vi "Durability Tank Cal UI.vi"(11 "Calling VI Ref":refnum<vi>) -> ()   [LabVIEW 2013]
uses:
  <vilib>/ptbypt/NI_PtbyPt.lvlib
  <vilib>/Utility/file.llb/Read From Spreadsheet File (string).vi
  <vilib>/Utility/miscctls.llb/LVRowAndColumnTypeDef.ctl
  <vilib>/Analysis/NI_AALPro.lvlib
  <resource>/objmgr/daqmx.rc
  Type Defs/Target Cluster Type Def.ctl
  Type Defs/Setpoint Cluster Type Def.ctl
  Type Defs/Targets Type Def.ctl
  <vilib>/Utility/config.llb/NI_LVConfig.lvlib
  Type Defs/Units Type Def (DAQ Rack).ctl
  Type Defs/Rack Version Type Def.ctl
  <userlib>/_OpenG.lib/array/array.llb/Remove Duplicates from 1D Array (DBL)__ogtk.vi
  <vilib>/Utility/file.llb/Write To Spreadsheet File (string).vi
  <vilib>/DAQmx/write.llb/DAQmx Write (Digital Bool 1Line 1Point).vi
  <vilib>/DAQmx/create/channels.llb/DAQmx Create Channel (DO-Digital Output).vi
  <vilib>/DAQmx/write.llb/DAQmx Write (Digital 1D Bool NChan 1Samp 1Line).vi
  <userlib>/_OpenG.lib/array/array.llb/Search 1D Array (String)__ogtk.vi
  Type Defs/System Type.ctl
  Type Defs/Registered System.ctl
  Type Defs/TCP Data Stream Mode (PC).ctl
  Type Defs/Channel Type Def (RIO).ctl
panel:
  in  "App Dir":path
  in  "Load Indicator Tab":enum32{"Page 1"}(tab)
  in  "Header Tab":enum32{"Page 1", "Page 2"}(tab)
  in  "Header OK":bool
  in  "Header Cancel":bool
  in  "Header Comments":string[][](table)=[["PRODUCT 5V. IS REFERENCE ONLY."], ["1"], ["2"]]
  in  "Cal Standards Table":string[][](table)=[["FLUKE MULTIMETER", "3539"], ["FLUKE CALIBRATOR", "7955"], ["", ""], ["", ""], ["", ""]]
  in  "Sys Cal Table":string[][](table)=[["CIB BD.", "DSS 9372-1"], ["D/A BD.", "DSS 9372-2"], ["", ""], ["", ""], ["", ""]]
  in  "Header Table 1":string[][](table)=[["9372blah"], ["DELPHI"], ["TL1181E"], ["EU2C397"], ["CIB/ D/A BD."], ["5 VOLTS"], ["NEW"], ["9087"]]
  in  "Header Table 2":string[][](table)=[["39687"], ["12"], ["40052"], ["MDC"], ["24"], ["48"], ["JUM  /   DR"]]
  in  "debug":bool=TRUE
  in  "Verify Tab":enum32{"Page 1", "Page 2"}(tab)
  in  "Hide Devs":bool
  in  "Auto":bool
  in  "Hide Cal Values":bool
  in  "Verify Edit":bool
  in  "Verify Table":string[][](table)=[["", "0", "0"], ["", "3", "3"], ["", "6", "6"], ["", "9", "9"], ["", "12", "12"], ["", "15", "15"], ["", "", ""], ["", "", ""], ["", "", ""], ["", "", ""]]
  in  "Verify Read":bool
  in  "ms":u32=1000
  in  "avg":i32=5
  in  "Output Tab":enum32{"Page 1", "Page 2"}(tab)
  out "Row":i32
  in  "Main Tab":enum32{"Page 1", "Page 2"}(tab)
  in  "Confirm 4th Point":bool
  out "Reading Value 4":dbl=0.001 caption="reading" format="%#.4g"
  in  "Cal Value 4":dbl caption="cal pt" format="%#.4g"
  in  "Confirm 5th Point":bool
  out "Reading Value 5":dbl=0.0016 caption="reading" format="%#.4g"
  in  "Cal Value 5":dbl caption="cal pt" format="%#.4g"
  in  "Start Verification":bool
  in  "View Spreadsheet":bool
  in  "Header":bool
  out "Cal Table":string[][](table)=[["AI-00", "V", "", "", "", "", "", "", "", "", "", "", "", "", "", "", "", "", "", "", "", "", "", "", "", "", "", "", "", "", "", ""], ["AI-01", "V", "", "", "", "", "", "", "", "", "", "", "", "", "", "", "", "", "", "", "", "", "", "", "", "", "", "", "", "", "", ""], ["AI-02", "V", "", "", "", "", "", "", "", "", "", "", "", "", "", "", "", "", "", "", "", "", "", "", "", "", "", "", "", "", "", ""], ["AI-03", "V", "", "", "", "", "", "", "", "", "", "", "", "", "", "", "", "", "", "", "", "", "", "", "", "", "", "", "", "", "", ""], ["AI-04", "V", "", "", "", "", "", "", "", "", "", "", "", "", "", "", "", "", "", "", "", "", "", "", "", "", "", "", "", "", "", ""], ["AI-05", "V", "", "", "", "", "", "", "", "", "", "", "", "", "", "", "", "", "", "", "", "", "", "", "", "", "", "", "", "", "", ""], ["AI-06", "V", "", "", "", "", "", "", "", "", "", "", "", "", "", "", "", "", "", "", "", "", "", "", "", "", "", "", "", "", "", ""], ["AI-07", "V", "", "", "", "", "", "", "", "", "", "", "", "", "", "", "", "", "", "", "", "", "", "", "", "", "", "", "", "", "", ""], ["AI-08", "V", "", "", "", "", "", "", "", "", "", "", "", "", "", "", "", "", "", "", "", "", "", "", "", "", "", "", "", "", "", ""], ["AI-09", "V", "", "", "", "", "", "", "", "", "", "", "", "", "", "", "", "", "", "", "", "", "", "", "", "", "", "", "", "", "", ""], ["AI-10", "V", "", "", "", "", "", "", "", "", "", "", "", "", "", "", "", "", "", "", "", "", "", "", "", "", "", "", "", "", "", ""], ["AI-11", "V", "", "", "", "", "", "", "", "", "", "", "", "", "", "", "", "", "", "", "", "", "", "", "", "", "", "", "", "", "", ""], ["AI-12", "V", "", "", "", "", "", "", "", "", "", "", "", "", "", "", "", "", "", "", "", "", "", "", "", "", "", "", "", "", "", ""], ["AI-13", "V", "", "", "", "", "", "", "", "", "", "", "", "", "", "", "", "", "", "", "", "", "", "", "", "", "", "", "", "", "", ""], ["AI-14", "V", "", "", "", "", "", "", "", "", "", "", "", "", "", "", "", "", "", "", "", "", "", "", "", "", "", "", "", "", "", ""], ["AI-15", "V", "", "", "", "", "", "", "", "", "", "", "", "", "", "", "", "", "", "", "", "", "", "", "", "", "", "", "", "", "", ""], ["AI-16", "V", "", "", "", "", "", "", "", "", "", "", "", "", "", "", "", "", "", "", "", "", "", "", "", "", "", "", "", "", "", ""], ["AI-17", "V", "", "", "", "", "", "", "", "", "", "", "", "", "", "", "", "", "", "", "", "", "", "", "", "", "", "", "", "", "", ""], ["AI-18", "V", "", "", "", "", "", "", "", "", "", "", "", "", "", "", "", "", "", "", "", "", "", "", "", "", "", "", "", "", "", ""], ["AI-19", "V", "", "", "", "", "", "", "", "", "", "", "", "", "", "", "", "", "", "", "", "", "", "", "", "", "", "", "", "", "", ""], ["AI-20", "V", "", "", "", "", "", "", "", "", "", "", "", "", "", "", "", "", "", "", "", "", "", "", "", "", "", "", "", "", "", ""], ["AI-21", "V", "", "", "", "", "", "", "", "", "", "", "", "", "", "", "", "", "", "", "", "", "", "", "", "", "", "", "", "", "", ""], ["AI-22", "V", "", "", "", "", "", "", "", "", "", "", "", "", "", "", "", "", "", "", "", "", "", "", "", "", "", "", "", "", "", ""], ["AI-23", "V", "", "", "", "", "", "", "", "", "", "", "", "", "", "", "", "", "", "", "", "", "", "", "", "", "", "", "", "", "", ""], ["AI-24", "V", "", "", "", "", "", "", "", "", "", "", "", "", "", "", "", "", "", "", "", "", "", "", "", "", "", "", "", "", "", ""], ["AI-25", "V", "", "", "", "", "", "", "", "", "", "", "", "", "", "", "", "", "", "", "", "", "", "", "", "", "", "", "", "", "", ""], ["AI-26", "V", "", "", "", "", "", "", "", "", "", "", "", "", "", "", "", "", "", "", "", "", "", "", "", "", "", "", "", "", "", ""], ["AI-27", "V", "", "", "", "", "", "", "", "", "", "", "", "", "", "", "", "", "", "", "", "", "", "", "", "", "", "", "", "", "", ""], ["AI-28", "V", "", "", "", "", "", "", "", "", "", "", "", "", "", "", "", "", "", "", "", "", "", "", "", "", "", "", "", "", "", ""], ["AI-29", "V", "", "", "", "", "", "", "", "", "", "", "", "", "", "", "", "", "", "", "", "", "", "", "", "", "", "", "", "", "", ""], ["AI-30", "V", "", "", "", "", "", "", "", "", "", "", "", "", "", "", "", "", "", "", "", "", "", "", "", "", "", "", "", "", "", ""], ["AI-31", "V", "", "", "", "", "", "", "", "", "", "", "", "", "", "", "", "", "", "", "", "", "", "", "", "", "", "", "", "", "", ""], ["TC-00", "degF", "", "", "", "", "", "", "", "", "", "", "", "", "", "", "", "", "", "", "", "", "", "", "", "", "", "", "", "", "", ""], ["TC-01", "degF", "", "", "", "", "", "", "", "", "", "", "", "", "", "", "", "", "", "", "", "", "", "", "", "", "", "", "", "", "", ""], ["TC-02", "degF", "", "", "", "", "", "", "", "", "", "", "", "", "", "", "", "", "", "", "", "", "", "", "", "", "", "", "", "", "", ""], ["TC-03", "degF", "", "", "", "", "", "", "", "", "", "", "", "", "", "", "", "", "", "", "", "", "", "", "", "", "", "", "", "", "", ""], ["TC-04", "degF", "", "", "", "", "", "", "", "", "", "", "", "", "", "", "", "", "", "", "", "", "", "", "", "", "", "", "", "", "", ""], ["TC-05", "degF", "", "", "", "", "", "", "", "", "", "", "", "", "", "", "", "", "", "", "", "", "", "", "", "", "", "", "", "", "", ""], ["TC-06", "degF", "", "", "", "", "", "", "", "", "", "", "", "", "", "", "", "", "", "", "", "", "", "", "", "", "", "", "", "", "", ""], ["TC-07", "degF", "", "", "", "", "", "", "", "", "", "", "", "", "", "", "", "", "", "", "", "", "", "", "", "", "", "", "", "", "", ""], ["TC-08", "degF", "", "", "", "", "", "", "", "", "", "", "", "", "", "", "", "", "", "", "", "", "", "", "", "", "", "", "", "", "", ""], ["TC-09", "degF", "", "", "", "", "", "", "", "", "", "", "", "", "", "", "", "", "", "", "", "", "", "", "", "", "", "", "", "", "", ""], ["TC-10", "degF", "", "", "", "", "", "", "", "", "", "", "", "", "", "", "", "", "", "", "", "", "", "", "", "", "", "", "", "", "", ""], ["TC-11", "degF", "", "", "", "", "", "", "", "", "", "", "", "", "", "", "", "", "", "", "", "", "", "", "", "", "", "", "", "", "", ""], ["TC-12", "degF", "", "", "", "", "", "", "", "", "", "", "", "", "", "", "", "", "", "", "", "", "", "", "", "", "", "", "", "", "", ""], ["TC-13", "degF", "", "", "", "", "", "", "", "", "", "", "", "", "", "", "", "", "", "", "", "", "", "", "", "", "", "", "", "", "", ""], ["TC-14", "degF", "", "", "", "", "", "", "", "", "", "", "", "", "", "", "", "", "", "", "", "", "", "", "", "", "", "", "", "", "", ""], ["TC-15", "degF", "", "", "", "", "", "", "", "", "", "", "", "", "", "", "", "", "", "", "", "", "", "", "", "", "", "", "", "", "", ""], ["", "", "", "", "", "", "", "", "", "", "", "", "", "", "", "", "", "", "", "", "", "", "", "", "", "", "", "", "", "", "", ""]]
  out "Tank IP:":string
  in  "Start Cal":bool
  in  "Confirm 1st Point":bool
  out "Reading Value 1":dbl caption="reading" format="%#.4g"
  in  "Cal Value 1":dbl caption="cal pt" format="%#.4g"
  in  "Confirm 2nd Point":bool
  out "Reading Value 2":dbl=0.001 caption="reading" format="%#.4g"
  in  "Cal Value 2":dbl caption="cal pt" format="%#.4g"
  in  "Save Cal":bool
  out "f(x)":dbl format="%#.4g"
  out "a0":dbl format="%#.4g"
  out "x":dbl=0.0006000000000000001 format="%#.4g"
  out "a2":dbl format="%#.4g"
  in  "Cancel Cal":bool
  out "Cal Unit":T1
  in  "Confirm 3rd Point":bool
  out "Reading Value 3":dbl=0.0016 caption="reading" format="%#.4g"
  in  "Cal Value 3":dbl caption="cal pt" format="%#.4g"
  out "a1":dbl format="%#.4g"
  in  "Channel to Cal":T2
  out "a3":dbl format="%#.4g"
  out "a4":dbl format="%#.4g"
  # "System Calibration Components"
  # "Calibration Standards Used"
  # "Output Control"
  # "1) Enter Header Info"
  # "3)  Select Channel to Calibrate"
  # "4) Start Procedure"
  # "-or-"
  # "5)  Take First Reading"
  # "6)  Take Second Reading"
  # "7)  Take Third Reading"
  # "8)  Take Fourth Reading"
  # "9)  Take Final Reading"
  # "10)  Review"
  # "11)  Confirm"
  # "Cal Spreadsheet"
  # "*Excel must be closed to return control to this app."
  # "2"
  # "3"
  # "4"
  # "x    +"
  # "x    +"
  # "x"
  # "="
  # "+"
  # "+"
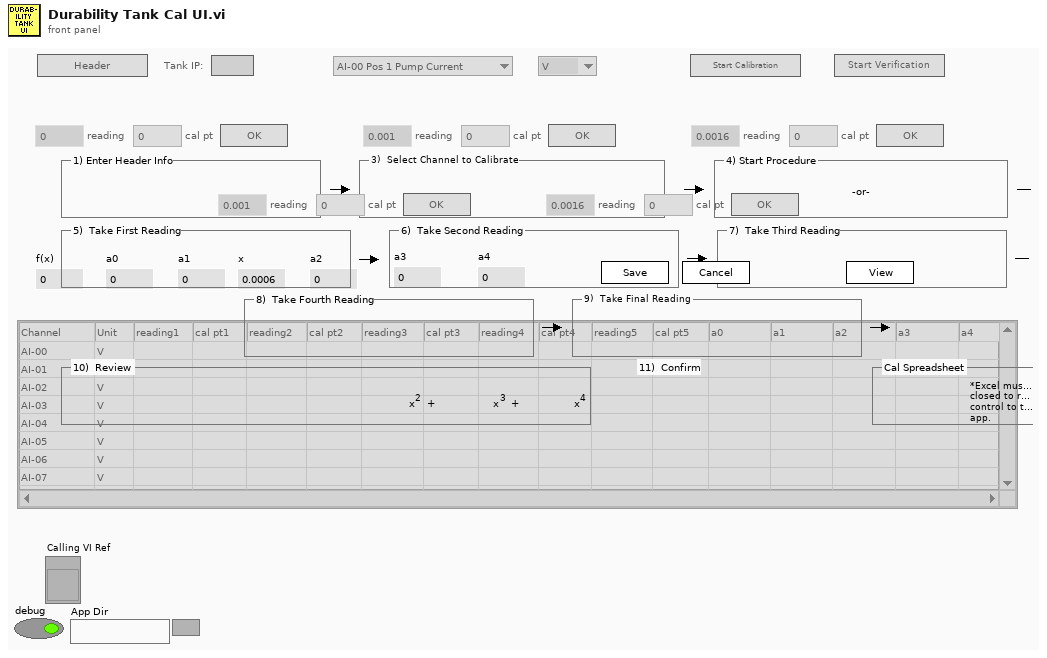
[diagram p1: front panel]
types:
  T1 = typedef "Units Type Def (DAQ Rack).ctl" = enum16{"V", "mA", "A", "Hz", "deg C"}
  T2 = typedef "Channel Type Def (RIO).ctl" = enum16{"AI-00 Pos 1 Pump Current", "AI-01 Pos 2 Pump Current", "AI-02 Pos 3 Pump Current", "AI-03 Pos 4 Pump Current", "AI-04 Pos 5 Pump Current", "AI-05 Pos 6 Pump Current", "AI-06 Pos 1 Speed", "AI-07 Pos 2 speed", "AI-08 Pos 3 Speed", "AI-09 Pos 4 Speed", "AI-10 Pos 5 Speed", "AI-11 Pos 6 Speed", "AI-12 Pos 1 Controller Current", "AI-13 Pos 2 Controller Current", "AI-14 Pos 3 Controller Current", "AI-15 Pos 4 Controller Current", "AI-16 Pos 5 Controller Current", "AI-17 Pos 6 Controller Current", "AI-18 Spare", "AI-19 Tank 1 Temperature", "AI-20 Tank 2 Temperature", "AI-21 Power Supply Voltage", "AI-22 Pos 1 Pressure", "AI-23 Pos 2 Pressure", "AI-24 Pos 3 Pressure", "AI-25 Pos 4 Pressure", "AI-26 Pos 5 Pressure", "AI-27 Pos 6 Pressure", "AI-28 Pos 1 Flow", "AI-29 Pos 2 Flow", "AI-30 Pos 3 Flow", "AI-31 Pos 4 Flow", "AI-32 Pos 5 Flow", "AI-33 Pos 6 Flow", "AI-34 Spare", "AI-35 Spare", "AI-36 Spare", "AI-37 Spare"}
  T3 = typedef "Registered System.ctl" = cluster{"System Type":T4, "Serial Number":string, "ID":string, "Cal File?":bool}
  T4 = typedef "System Type.ctl" = enum16{"DAQ Rack", "DAQ Cart", "RIO", "cDAQ", "unknown", "open"}
  T5 = typedef "Rack Version Type Def.ctl" = enum16{"Volts & TC", "Volts", "RIO", "cDAQ", "Volts & Current", "Cart"}
  T6 = typedef "Targets Type Def.ctl" = cluster{"V Targets":T7, "5V Targets":T7, "mA Targets":T7, "A Targets":T7, "Hz Targets":T7, "TC Targets":T7, "V Setpoints":T8, "5V Setpoints":T8, "mA Setpoints ":T8, "A Setpoints":T8, "Hz Setpoints":T8, "25A Setpoints":T8, "25A Targets":T7, "CT Targets":T7, "DegC Targets":T7, "kPa Targets":T7, "LpH Targets":T7, "CT Setpoints":T8, "DegC Setpoints":T8, "kPa Setpoints":T8, "LpH Setpoints":T8}
  T7 = typedef "Target Cluster Type Def.ctl" = cluster{"target1":dbl, "target2":dbl, "target3":dbl, "target4":dbl, "target5":dbl, "target6":dbl, "target7":dbl, "target8":dbl, "target9":dbl, "target10":dbl}
  T8 = typedef "Setpoint Cluster Type Def.ctl" = cluster{"setpoint1":dbl, "setpoint2":dbl, "setpoint3":dbl, "setpoint4":dbl, "setpoint5":dbl}
  T9 = cluster{"Error":errorcluster, "Cal Log":string[][], "Cal Log Header":string[], "Cal Files Base Path":path, "Default Cal Log":string[][], "Samples to Avg":i32, "Base Path":path, "Cal Targets Path":path, "Calling VI Ref":refnum<vi>, "Selected Chassis":tag, "debug":bool, "Verify Table":string[][], "Cal Template Path":path, "Cal Spreadsheet Path":path, "Verify Table Ref":refnum<vi>, "Init Mean":bool, "Auto":bool, "App Dir":path, "DAQ Rack":string, "Cal File Path":path, "Targets":T6, "Cal Unit":T1, "Channel to Cal":T2, "Rack Version":T5, "Verification":bool, "Registered Systems":T3[], "Desired System":T3, "Cal Target Array":string[]}
  T10 = enum8{"Enabled", "Disabled", "Disabled and Grayed Out"}
  T11 = typedef "LVRowAndColumnTypeDef.ctl" = cluster{"Row":i32, "Column":i32}
  T12 = typedef "TCP Data Stream Mode (PC).ctl" = enum16{"Init", "Read Data", "Close"}
  T13 = enum32{"Bad", "Idle", "Run top level", "Running"}
  T14 = cluster{"[0]":dbl, "[1]":dbl, "[2]":dbl, "[3]":dbl, "[4]":dbl, "[5]":dbl, "[6]":dbl, "[7]":dbl, "[8]":dbl, "[9]":dbl}
  T15 = typedef "NI_LVConfig.lvlib/Config Data RefNum.ctl" = refnum<k1>
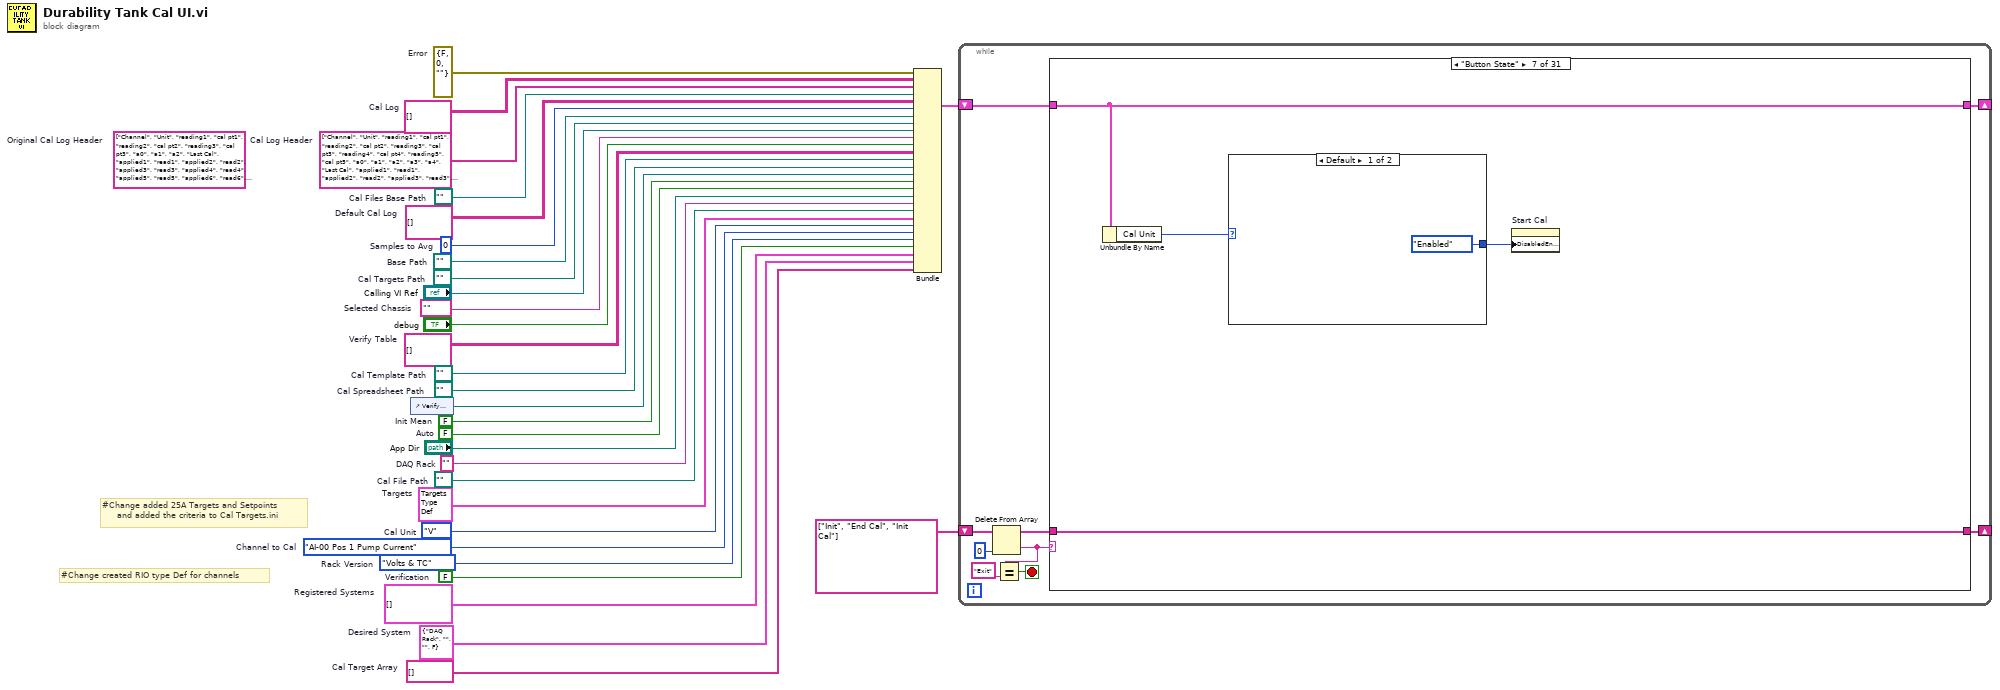
[diagram p0: block diagram]
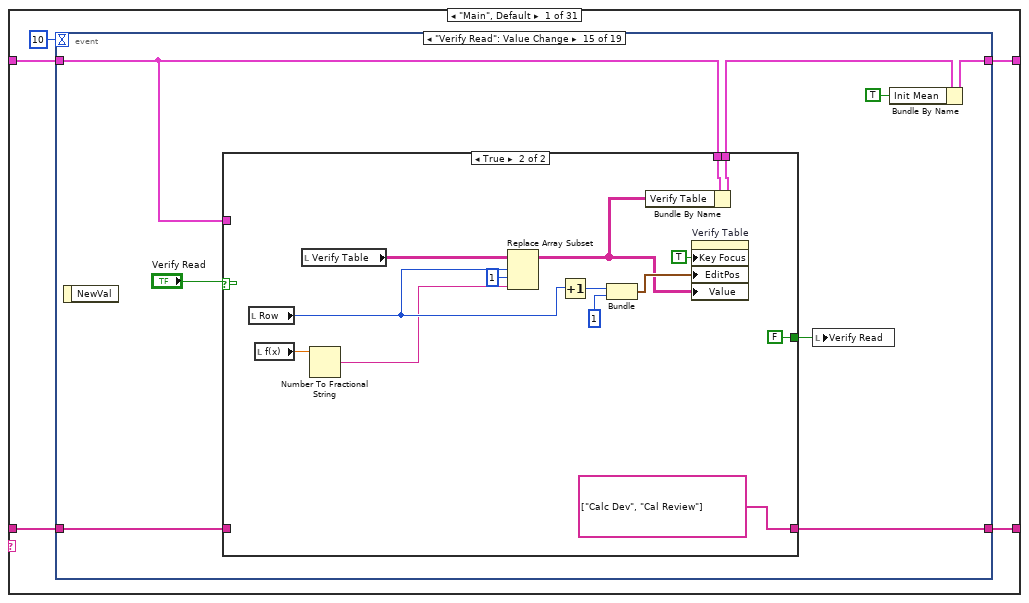
[diagram p2: hidden frame]
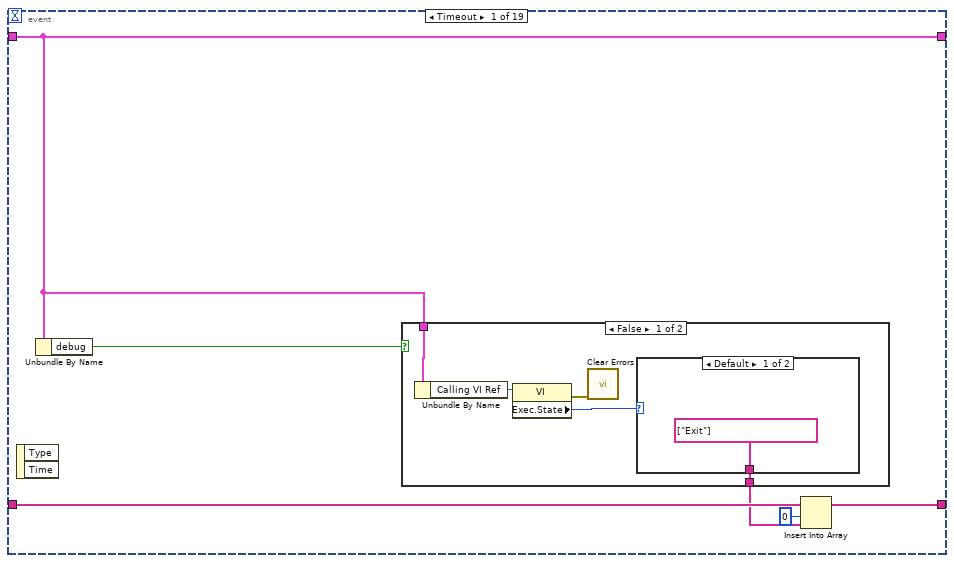
[diagram p3: hidden frame]
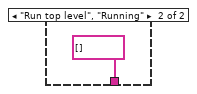
[diagram p4: hidden frame]
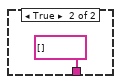
[diagram p5: hidden frame]
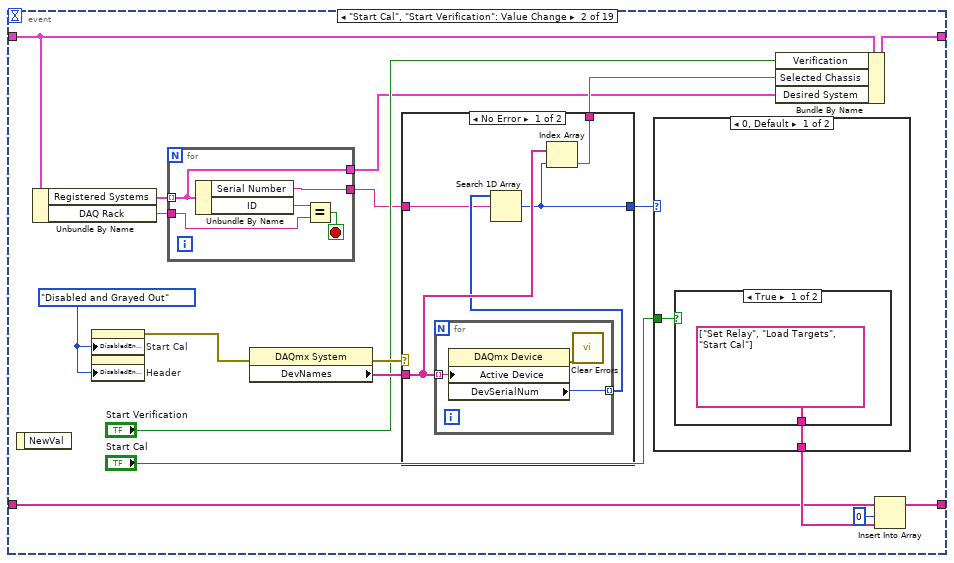
[diagram p6: hidden frame]
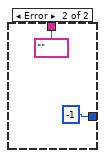
[diagram p7: hidden frame]
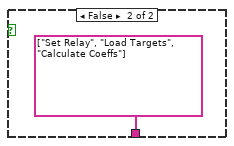
[diagram p8: hidden frame]
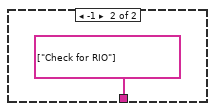
[diagram p9: hidden frame]
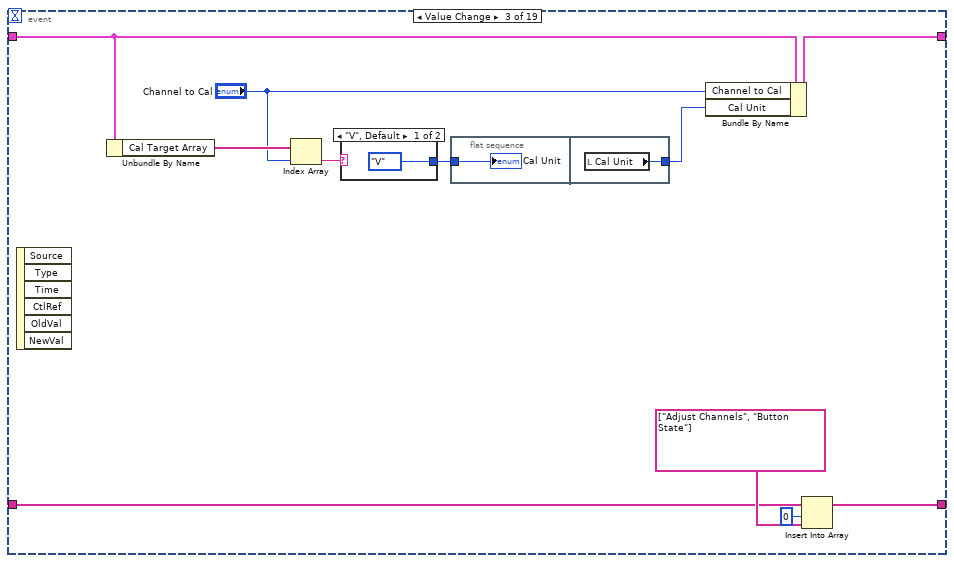
[diagram p10: hidden frame]
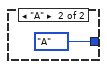
[diagram p11: hidden frame]
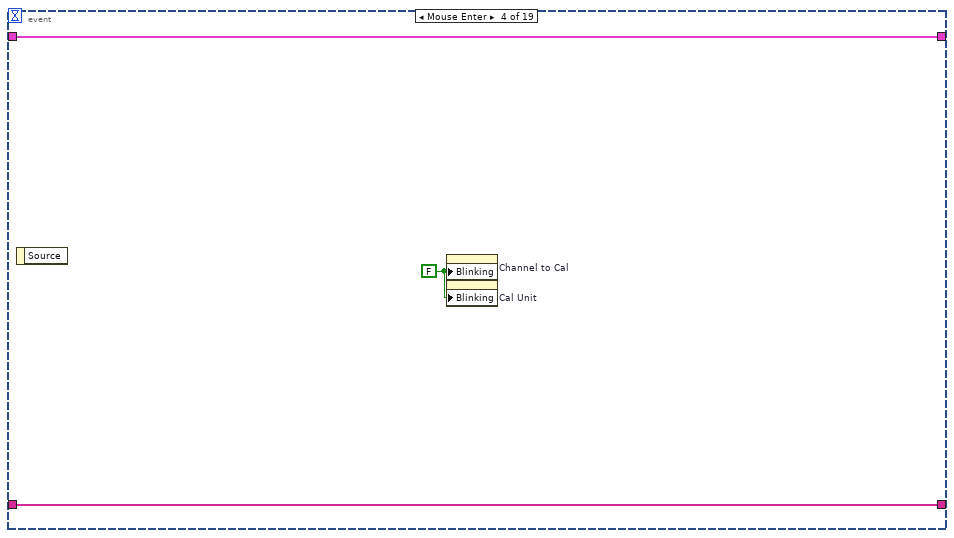
[diagram p12: hidden frame]
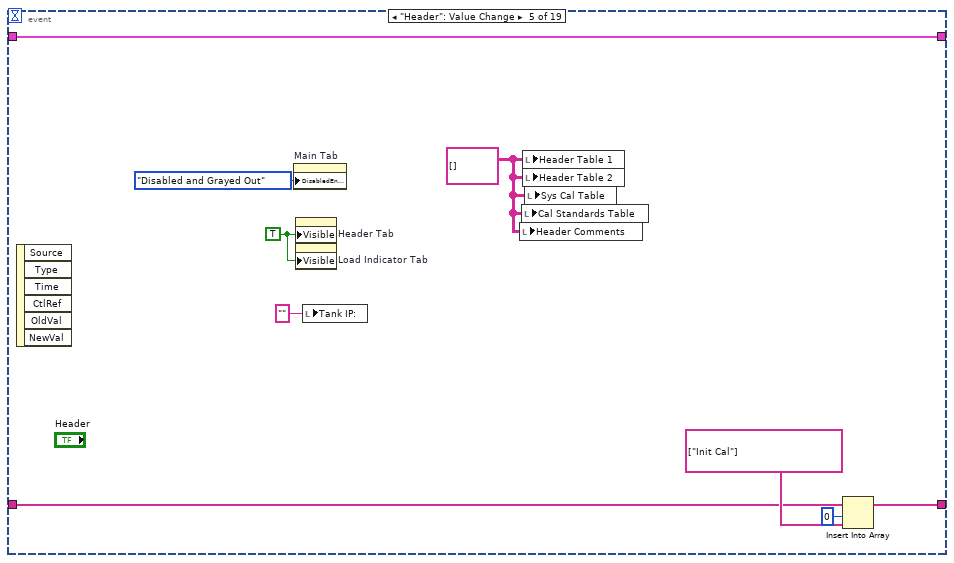
[diagram p13: hidden frame]
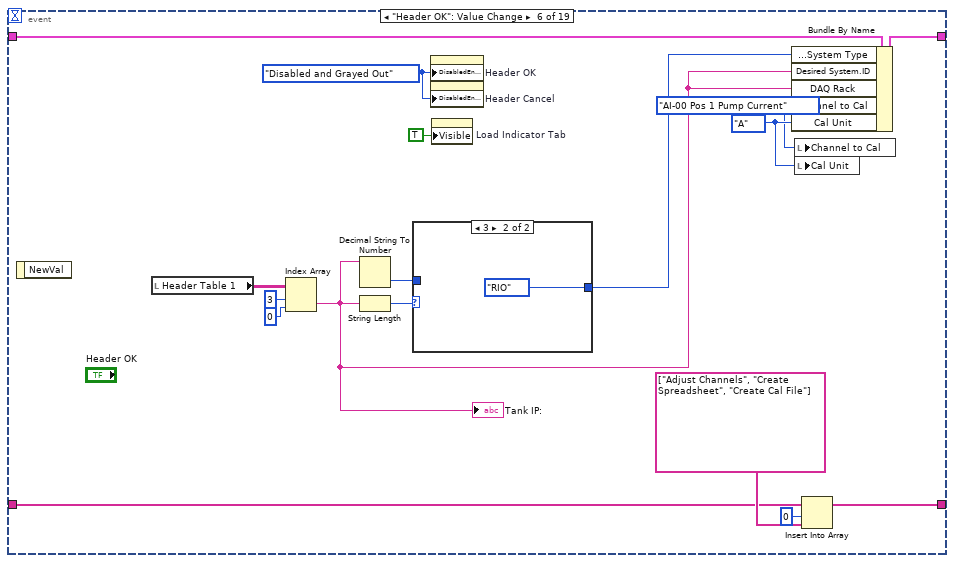
[diagram p14: hidden frame]
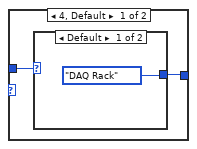
[diagram p15: hidden frame]
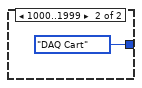
[diagram p16: hidden frame]
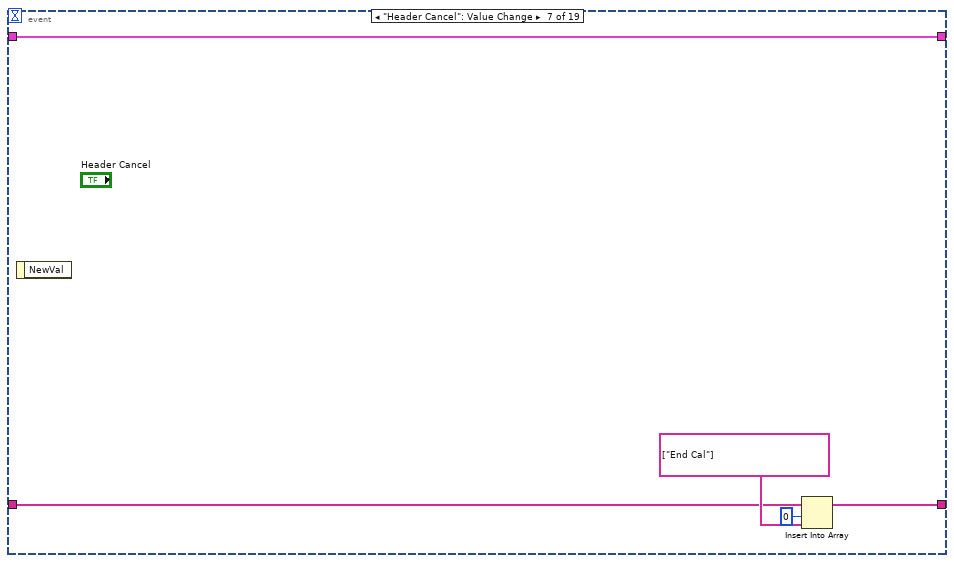
[diagram p17: hidden frame]
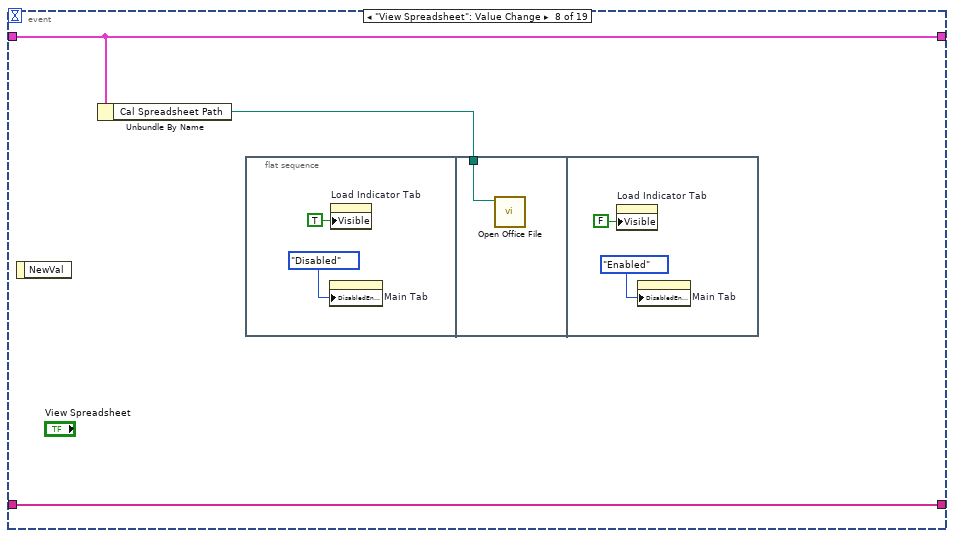
[diagram p18: hidden frame]
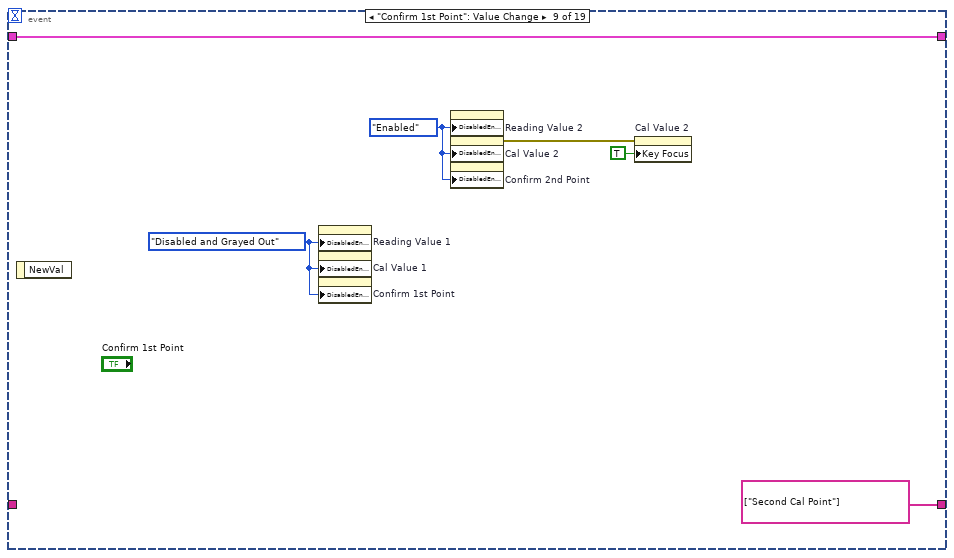
[diagram p19: hidden frame]
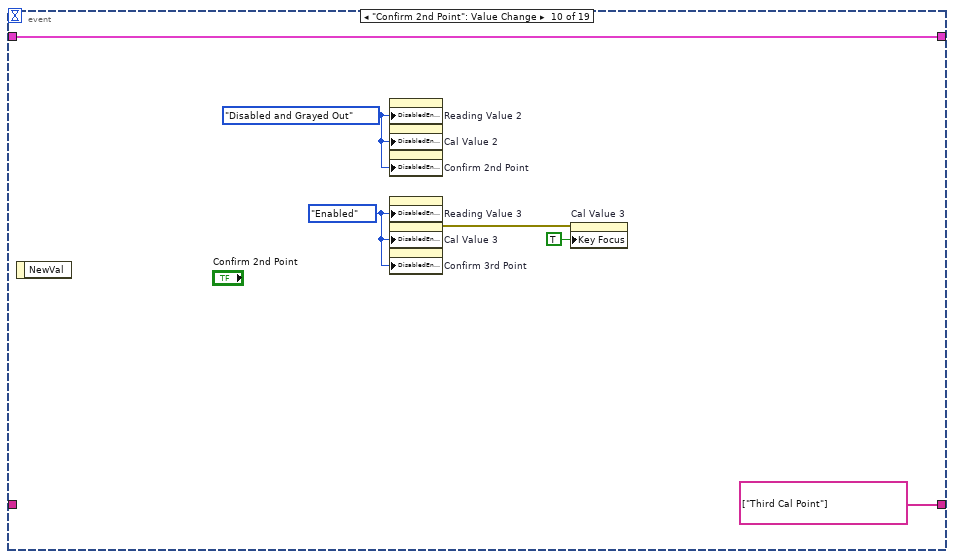
[diagram p20: hidden frame]
diagram:
  w1 = string[] ["Channel", "Unit", "reading1", "cal pt1", "reading2", "cal pt2", "reading3", "cal pt3", "reading4", "cal pt4", "reading5", "cal pt5", "a0", "a1", "a2", "a3", "a4", "Last Cal", "applied1", "read1", "applied2", "read2", "applied3", "read3", "applied4", "read4", "applied5", "read5", "applied6", "read6", "applied7", "read7", "applied8", "read8", "applied9", "read9", "applied10", "read10"]  # Cal Log Header
  w2 = string[] []  # Cal Target Array
  w3 = Channel_Type_Def_(RIO)."AI-00 Pos 1 Pump Current"  # Channel to Cal
  w4 = T3 {"System Type"=enum."DAQ Rack", "Serial Number"="", "ID"="", "Cal File?"=FALSE}  # Desired System
  w5 = T3[] []  # Registered Systems
  w6 = FALSE  # Verification
  w7 = Rack_Version_Type_Def."Volts & TC"  # Rack Version
  w8 = Units_Type_Def_(DAQ_Rack)."V"  # Cal Unit
  w9 = T6 {"V Targets"={"target1"=0.0, "target2"=0.0, "target3"=0.0, "target4"=0.0, "target5"=0.0, "target6"=0.0, "target7"=0.0, "target8"=0.0, "target9"=0.0, "target10"=0.0}, "5V Targets"={"target1"=0.0, "target2"=0.0, "target3"=0.0, "target4"=0.0, "target5"=0.0, "target6"=0.0, "target7"=0.0, "target8"=0.0, "target9"=0.0, "target10"=0.0}, "mA Targets"={"target1"=0.0, "target2"=0.0, "target3"=0.0, "target4"=0.0, "target5"=0.0, "target6"=0.0, "target7"=0.0, "target8"=0.0, "target9"=1.0, "target10"=0.0}, "A Targets"={"target1"=0.0, "target2"=0.0, "target3"=0.0, "target4"=0.0, "target5"=0.0, "target6"=0.0, "target7"=0.0, "target8"=0.0, "target9"=0.0, "target10"=0.0}, "Hz Targets"={"target1"=0.0, "target2"=0.0, "target3"=0.0, "target4"=0.0, "target5"=0.0, "target6"=0.0, "target7"=0.0, "target8"=0.0, "target9"=0.0, "target10"=0.0}, "TC Targets"={"target1"=0.0, "target2"=0.0, "target3"=0.0, "target4"=0.0, "target5"=0.0, "target6"=0.0, "target7"=0.0, "target8"=0.0, "target9"=0.0, "target10"=0.0}, "V Setpoints"={"setpoint1"=0.0, "setpoint2"=0.0, "setpoint3"=0.0, "setpoint4"=0.0, "setpoint5"=0.0}, "5V Setpoints"={"setpoint1"=0.0, "setpoint2"=0.0, "setpoint3"=0.0, "setpoint4"=0.0, "setpoint5"=0.0}, "mA Setpoints "={"setpoint1"=0.0, "setpoint2"=0.0, "setpoint3"=0.0, "setpoint4"=0.0, "setpoint5"=0.0}, "A Setpoints"={"setpoint1"=0.0, "setpoint2"=0.0, "setpoint3"=0.0, "setpoint4"=0.0, "setpoint5"=0.0}, "Hz Setpoints"={"setpoint1"=0.0, "setpoint2"=0.0, "setpoint3"=0.0, "setpoint4"=0.0, "setpoint5"=0.0}, "25A Setpoints"={"setpoint1"=0.0, "setpoint2"=0.0, "setpoint3"=0.0, "setpoint4"=0.0, "setpoint5"=0.0}, "25A Targets"={"target1"=0.0, "target2"=0.0, "target3"=0.0, "target4"=0.0, "target5"=0.0, "target6"=0.0, "target7"=0.0, "target8"=0.0, "target9"=0.0, "target10"=0.0}, "CT Targets"={"target1"=0.0, "target2"=0.0, "target3"=0.0, "target4"=0.0, "target5"=0.0, "target6"=0.0, "target7"=0.0, "target8"=0.0, "target9"=0.0, "target10"=0.0}, "DegC Targets"={"target1"=0.0, "target2"=0.0, "target3"=0.0, "target4"=0.0, "target5"=0.0, "target6"=0.0, "target7"=0.0, "target8"=0.0, "target9"=0.0, "target10"=0.0}, "kPa Targets"={"target1"=0.0, "target2"=0.0, "target3"=0.0, "target4"=0.0, "target5"=0.0, "target6"=0.0, "target7"=0.0, "target8"=0.0, "target9"=0.0, "target10"=0.0}, "LpH Targets"={"target1"=0.0, "target2"=0.0, "target3"=0.0, "target4"=0.0, "target5"=0.0, "target6"=0.0, "target7"=0.0, "target8"=0.0, "target9"=0.0, "target10"=0.0}, "CT Setpoints"={"setpoint1"=0.0, "setpoint2"=0.0, "setpoint3"=0.0, "setpoint4"=0.0, "setpoint5"=0.0}, "DegC Setpoints"={"setpoint1"=0.0, "setpoint2"=0.0, "setpoint3"=0.0, "setpoint4"=0.0, "setpoint5"=0.0}, "kPa Setpoints"={"setpoint1"=0.0, "setpoint2"=0.0, "setpoint3"=0.0, "setpoint4"=0.0, "setpoint5"=0.0}, "LpH Setpoints"={"setpoint1"=0.0, "setpoint2"=0.0, "setpoint3"=0.0, "setpoint4"=0.0, "setpoint5"=0.0}}  # Targets
  w10 = path ""  # Cal File Path
  w11 = ""  # DAQ Rack
  w13 = FALSE  # Auto
  w14 = FALSE  # Init Mean
  w16 = path ""  # Cal Spreadsheet Path
  w17 = path ""  # Cal Template Path
  w18 = string[][] []  # Verify Table
  w20 = tag ""  # Selected Chassis
  w22 = path ""  # Cal Targets Path
  w23 = path ""  # Base Path
  w25 = 0  # Samples to Avg
  w26 = string[][] []  # Default Cal Log
  w27 = path ""  # Cal Files Base Path
  (unwired) string[] ["Channel", "Unit", "reading1", "cal pt1", "reading2", "cal pt2", "reading3", "cal pt3", "a0", "a1", "a2", "Last Cal", "applied1", "read1", "applied2", "read2", "applied3", "read3", "applied4", "read4", "applied5", "read5", "applied6", "read6", "applied7", "read7", "applied8", "read8", "applied9", "read9", "applied10", "read10"]  # Original Cal Log Header
  w28 = string[][] []  # Cal Log
  w24 = errorcluster {"status"=FALSE, "code"=0, "source"=""}  # Error
  # "#Change created RIO type Def for channels"
  # "#Change added 25A Targets and Setpoints\n     and added the criteria to Cal Targets.ini"
  n1 = control-ref of="Verify Table Ref"() -> (w15:refnum<vi>)
  n2 = Bundle("Error"=w24, "Cal Log"=w28, "Cal Log Header"=w1, "Cal Files Base Path"=w27, "Default Cal Log"=w26, "Samples to Avg"=w25, "Base Path"=w23, "Cal Targets Path"=w22, "Calling VI Ref"="Calling VI Ref", "Selected Chassis"=w20, "debug"="debug", "Verify Table"=w18, "Cal Template Path"=w17, "Cal Spreadsheet Path"=w16, "Verify Table Ref"=w15, "Init Mean"=w14, "Auto"=w13, "App Dir"="App Dir", "DAQ Rack"=w11, "Cal File Path"=w10, "Targets"=w9, "Cal Unit"=w8, "Channel to Cal"=w3, "Rack Version"=w7, "Verification"=w6, "Registered Systems"=w5, "Desired System"=w4, "Cal Target Array"=w2) -> (w29:T9)  [unwired: 1 in]
  n3 = while {
    shift-right: [w31] -> _
    shift-left: string[] ["Init", "End Cal", "Init Cal"] -> [w39]
    shift-right: [w33] -> _
    shift-left: w29 -> [w34]
    stop <- w38 stop-if-true
    n4 = Delete From Array(array=w39, index=0) -> (deleted portion=w36:string, array with subset deleted=w37:string[])  [unwired: 1 in]
    n5 = Equal?(x=w36, y="Exit" ("x")) -> (x = y?=w38:bool)
    n6 = case shown="\"Button State\"" w36 {
      tunnel: w37 -> [w43 w286 w300 w307 w322 w346 w526 w532 w535 w539 w569 w605 w632 w656 w739 w762 w778 w792 w818 w844 w870 w896 w929 w1027 w1114 w1136 w1147 w1170 w1197 w1203 w1205]
      tunnel: w34 -> [w41 w278 w301 w314 w316 w344 w525 w531 w534 w537 w572 w607 w626 w654 w721 w761 w774 w790 w816 w842 w868 w894 w919 w1009 w1075 w1134 w1145 w1167 w1192 w1201 w1204]
      tunnel: [w40 w289 w301 w313 w316 w343 w525 w530 w534 w537 w571 w607 w625 w658 w735 w761 w774 w790 w816 w842 w868 w894 w919 w1004 w1075 w1133 w1145 w1167 w1192 w1202 w1204] -> w33
      tunnel: [w42 w286 w300 w304 w321 w346 w526 w532 w535 w538 w570 w606 w633 w657 w739 w762 w779 w793 w817 w843 w869 w895 w930 w1028 w1115 w1135 w1146 w1170 w1198 w1203 w1205] -> w31
      frame "Main", Default {
        n7 = event shown="[14] \"Verify Read\": Value Change" {
          selector: _ -> [_ _ _ _ _ _ _ _ _ _ _ _ _ _ _ _ _ _ _]
          dyn-events: _ -> [_ _ _ _ _ _ _ _ _ _ _ _ _ _ _ _ _ _ _]
          timeout: 10 -> [_ _ _ _ _ _ _ _ _ _ _ _ _ _ _ _ _ _ _]
          tunnel: [w50 w75 w103 w113 w117 w137 w148 w153 string[] ["Second Cal Point"] string[] ["Third Cal Point"] string[] ["Fourth Cal Point"] string[] ["Final Cal Point"] string[] ["Calculate Coeffs"] string[] ["End Cal"] w188 w212 string[] ["Save Cal"] w255 string[] ["Calc Dev", "Cal Review"]] -> w42
          tunnel: w43 -> [w49 w74 w104 w113 w118 w136 w149 w153 _ _ _ _ _ _ w187 w212 _ w255 _]
          tunnel: [w47 w70 w107 w114 w123 w130 w147 w151 w160 w166 w176 w177 w183 w185 w190 w214 w249 w253 w262] -> w40
          tunnel: w41 -> [w47 w71 w102 w114 w123 w131 w147 w151 w160 w166 w176 w177 w183 w185 w192 w214 w249 w254 w263]
          event Timeout {
            n8 = event-data() -> ()  [unwired: 1 in, 2 out]
            n9 = Unbundle By Name(w47) -> ("debug"=w46:bool)
            n10 = case shown="False" w46 {
              tunnel: [w55 string[] []] -> w48
              tunnel: w47 -> [w52 _]
              frame False {
                n11 = Unbundle By Name(w52) -> ("Calling VI Ref"=w54:refnum<vi>)
                n12 = property class="VI"(reference=w54) -> (error out=w51:errorcluster, "Exec.State"=w53:T13)  [unwired: 1 in, 1 out]
                n13 = call <vilib>:"Clear Errors.vi"("error in (no error)"=w51) -> ()  [unwired: 6 in, 1 out]
                n14 = case shown="Default" w53 {
                  tunnel: [string[] ["Exit"] string[] []] -> w55
                  frame Default {
                  }
                  frame "Run top level", "Running" {
                  }
                }
              }
              frame True {
              }
            }
            n15 = Insert Into Array(array=w49, index=0, new element=w48) -> (w50:string[])
          }
          event "Start Cal", "Start Verification": Value Change {
            w66 = T10."Disabled and Grayed Out" ("Disabled")
            n16 = event-data() -> ()  [unwired: 1 in, 1 out]
            n17 = Unbundle By Name(w71) -> ("Registered Systems"=w62:T3[], "DAQ Rack"=w61:string)
            n18 = property on="Start Cal" class="Bool"("DisabledEnum"=w66) -> (error out=w65:errorcluster)  [unwired: 2 in, 1 out]
            n19 = property on="Header" class="Bool"("DisabledEnum"=w66) -> ()  [unwired: 2 in, 2 out]
            n20 = for {
              tunnel: w62 -> [w77] mode=indexing
              tunnel: w61 -> [w80]
              tunnel: [w78] -> w60
              tunnel: [w77] -> w59
              stop <- w79 stop-if-true
              n21 = Unbundle By Name(w77) -> ("Serial Number"=w78:string, "ID"=w81:string)
              n22 = Equal?(x=w81, y=w80) -> (x = y?=w79:bool)
            }
            n23 = property class="DAQmx System"(error in=w65) -> (error out=w68:errorcluster, "DevNames"=w73:tag[])  [unwired: 1 in, 1 out]
            n24 = case shown="No Error" w68 {
              tunnel: w60 -> [w82 _]
              tunnel: w73 -> [w86 _]
              tunnel: [w85 -1 ("index of element")] -> w72
              tunnel: [w84 tag ""] -> w69
              frame No Error {
                n25 = for {
                  tunnel: w86 -> [w89] mode=indexing
                  tunnel: [w88] -> w83 mode=indexing
                  n26 = property class="DAQmx Device"("Active Device"=w89) -> (error out=w87:errorcluster, "DevSerialNum"=w88:u32)  [unwired: 2 in, 1 out]
                  n27 = call <vilib>:"Clear Errors.vi"("error in (no error)"=w87) -> ()  [unwired: 6 in, 1 out]
                }
                n28 = Search 1D Array(1D array=w83, element=w82) -> (index of element=w85:i32)  [unwired: 1 in]
                n29 = Index Array(array=w86, index=w85) -> (element=w84:tag)
              }
              frame Error {
              }
            }
            n30 = case shown="0, Default" w72 {
              tunnel: [w93 string[] ["Check for RIO"]] -> w76
              tunnel: "Start Cal" -> [w92 _]
              frame 0, Default {
                n31 = case shown="True" w92 {
                  tunnel: [string[] ["Set Relay", "Load Targets", "Start Cal"] string[] ["Set Relay", "Load Targets", "Calculate Coeffs"]] -> w93
                  frame True {
                  }
                  frame False {
                  }
                }
              }
              frame -1 {
              }
            }
            n32 = Bundle By Name(cluster=w71, "Verification"="Start Verification", "Selected Chassis"=w69, "Desired System"=w59) -> (w70:T9)
            n33 = Insert Into Array(array=w74, index=0, new element=w76) -> (w75:string[])
          }
          event Value Change {
            n34 = event-data() -> ()  [unwired: 1 in, 6 out]
            n35 = Unbundle By Name(w102) -> ("Cal Target Array"=w101:string[])
            n36 = Index Array(array=w101, index="Channel to Cal") -> (element=w100:string)
            n37 = case shown="\"V\", Default" w100 {
              tunnel: [Units_Type_Def_(DAQ_Rack)."V" ("Cal Unit") Units_Type_Def_(DAQ_Rack)."A" ("Cal Unit")] -> w98
              frame "V", Default {
              }
              frame "A" {
              }
            }
            n38 = flat-sequence {
              tunnel: w98 -> [w110]
              tunnel: [w111] -> w97
              frame #0 {
                "Cal Unit" <- w110
              }
              frame #1 {
                n39 = local read "Cal Unit"() -> (w111:T1)
              }
            }
            n40 = Bundle By Name(cluster=w102, "Channel to Cal"="Channel to Cal", "Cal Unit"=w97) -> (w107:T9)
            n41 = Insert Into Array(array=w104, index=0, new element=string[] ["Adjust Channels", "Button State"]) -> (w103:string[])
          }
          event Mouse Enter {
            w112 = FALSE ("Blinking")
            n42 = event-data() -> ()  [unwired: 1 in, 1 out]
            n43 = property on="Channel to Cal" class="Enum (strict)"("Blinking"=w112) -> ()  [unwired: 2 in, 2 out]
            n44 = property on="Cal Unit" class="Enum (strict)"("Blinking"=w112) -> ()  [unwired: 2 in, 2 out]
          }
          event "Header": Value Change {
            w121 = string[][] [] ("Header Table 1")
            w120 = TRUE ("Visible")
            n45 = event-data() -> ()  [unwired: 1 in, 6 out]
            n46 = property on="Main Tab" class="TabCtl (strict)"("DisabledEnum"=T10."Disabled and Grayed Out" ("Disabled")) -> ()  [unwired: 2 in, 2 out]
            n47 = property on="Header Tab" class="TabCtl (strict)"("Visible"=w120) -> ()  [unwired: 2 in, 2 out]
            n48 = property on="Load Indicator Tab" class="TabCtl (strict)"("Visible"=w120) -> ()  [unwired: 2 in, 2 out]
            n49 = local write "Tank IP:"("" ("DAQ Rack")) -> ()
            n50 = local write "Header Comments"(w121) -> ()
            n51 = local write "Cal Standards Table"(w121) -> ()
            n52 = local write "Header Table 1"(w121) -> ()
            n53 = local write "Header Table 2"(w121) -> ()
            n54 = local write "Sys Cal Table"(w121) -> ()
            n55 = Insert Into Array(array=w118, index=0, new element=string[] ["Init Cal"]) -> (w117:string[])
          }
          event "Header OK": Value Change {
            w124 = Channel_Type_Def_(RIO)."AI-00 Pos 1 Pump Current" ("Channel to Cal")
            w129 = Units_Type_Def_(DAQ_Rack)."A" ("Cal Unit")
            w140 = T10."Disabled and Grayed Out" ("Disabled")
            n56 = event-data() -> ()  [unwired: 1 in, 1 out]
            n57 = local read "Header Table 1"() -> (w134:string[][])
            n58 = Index Array(array=w134, index (row)=3, index (col)=0 ("disabled index (col)")) -> (element=w126:string)
            "Tank IP:" <- w126
            n59 = Decimal String To Number(string=w126) -> (number=w125:i32)  [unwired: 2 in, 1 out]
            n60 = String Length(string=w126) -> (length=w128:i32)
            n61 = case shown="3" w128 {
              tunnel: [w141 System_Type."RIO" ("Desired System.System Type")] -> w127
              tunnel: w125 -> [w142 _]
              frame 4, Default {
                n62 = case shown="Default" w142 {
                  tunnel: [System_Type."DAQ Rack" ("Desired System.System Type") System_Type."DAQ Cart" ("Desired System.System Type")] -> w141
                  frame Default {
                  }
                  frame 1000..1999 {
                  }
                }
              }
              frame 3 {
              }
            }
            n63 = property on="Header OK" class="Bool"("DisabledEnum"=w140) -> ()  [unwired: 2 in, 2 out]
            n64 = property on="Header Cancel" class="Bool"("DisabledEnum"=w140) -> ()  [unwired: 2 in, 2 out]
            n65 = property on="Load Indicator Tab" class="TabCtl (strict)"("Visible"=TRUE) -> ()  [unwired: 2 in, 2 out]
            n66 = Bundle By Name(cluster=w131, "Desired System.System Type"=w127, "Desired System.ID"=w126, "DAQ Rack"=w126, "Channel to Cal"=w124, "Cal Unit"=w129) -> (w130:T9)
            n67 = local write "Channel to Cal"(w124) -> ()
            n68 = local write "Cal Unit"(w129) -> ()
            n69 = Insert Into Array(array=w136, index=0, new element=string[] ["Adjust Channels", "Create Spreadsheet", "Create Cal File"]) -> (w137:string[])
          }
          event "Header Cancel": Value Change {
            n70 = event-data() -> ()  [unwired: 1 in, 1 out]
            n71 = Insert Into Array(array=w149, index=0, new element=string[] ["End Cal"]) -> (w148:string[])
          }
          event "View Spreadsheet": Value Change {
            n72 = event-data() -> ()  [unwired: 1 in, 1 out]
            n73 = Unbundle By Name(w151) -> ("Cal Spreadsheet Path"=w152:path)
            n74 = flat-sequence {
              tunnel: w152 -> [w156]
              frame #0 {
                n75 = property on="Main Tab" class="TabCtl (strict)"("DisabledEnum"=T10."Disabled" ("Disabled")) -> ()  [unwired: 2 in, 2 out]
                n76 = property on="Load Indicator Tab" class="TabCtl (strict)"("Visible"=TRUE) -> ()  [unwired: 2 in, 2 out]
              }
              frame #1 {
                n77 = call "Open Office File.vi"("Selection a Word (.doc, .docx), Excel (.xls, .xlsx), or Powerpoint (.ppt, .pptx) Document..."=w156) -> ()  [unwired: 10 in, 1 out]
              }
              frame #2 {
                n78 = property on="Load Indicator Tab" class="TabCtl (strict)"("Visible"=FALSE) -> ()  [unwired: 2 in, 2 out]
                n79 = property on="Main Tab" class="TabCtl (strict)"("DisabledEnum"=T10."Enabled" ("Disabled")) -> ()  [unwired: 2 in, 2 out]
              }
            }
          }
          event "Confirm 1st Point": Value Change {
            w162 = T10."Disabled and Grayed Out" ("Disabled")
            w163 = T10."Enabled" ("Disabled")
            n80 = event-data() -> ()  [unwired: 1 in, 1 out]
            n81 = property on="Reading Value 1" class="DigNum (strict)"("DisabledEnum"=w162) -> ()  [unwired: 2 in, 2 out]
            n82 = property on="Cal Value 1" class="DigNum (strict)"("DisabledEnum"=w162) -> ()  [unwired: 2 in, 2 out]
            n83 = property on="Confirm 1st Point" class="Bool"("DisabledEnum"=w162) -> ()  [unwired: 2 in, 2 out]
            n84 = property on="Reading Value 2" class="DigNum (strict)"("DisabledEnum"=w163) -> ()  [unwired: 2 in, 2 out]
            n85 = property on="Cal Value 2" class="DigNum (strict)"("DisabledEnum"=w163) -> (error out=w161:errorcluster)  [unwired: 2 in, 1 out]
            n86 = property on="Confirm 2nd Point" class="Bool"("DisabledEnum"=w163) -> ()  [unwired: 2 in, 2 out]
            n87 = property on="Cal Value 2" class="DigNum (strict)"(error in=w161, "Key Focus"=TRUE) -> ()  [unwired: 1 in, 2 out]
          }
          event "Confirm 2nd Point": Value Change {
            w169 = T10."Enabled" ("Disabled")
            w170 = T10."Disabled and Grayed Out" ("Disabled")
            n88 = event-data() -> ()  [unwired: 1 in, 1 out]
            n89 = property on="Reading Value 2" class="DigNum (strict)"("DisabledEnum"=w170) -> ()  [unwired: 2 in, 2 out]
            n90 = property on="Cal Value 2" class="DigNum (strict)"("DisabledEnum"=w170) -> ()  [unwired: 2 in, 2 out]
            n91 = property on="Confirm 2nd Point" class="Bool"("DisabledEnum"=w170) -> ()  [unwired: 2 in, 2 out]
            n92 = property on="Reading Value 3" class="DigNum (strict)"("DisabledEnum"=w169) -> ()  [unwired: 2 in, 2 out]
            n93 = property on="Cal Value 3" class="DigNum (strict)"("DisabledEnum"=w169) -> (error out=w167:errorcluster)  [unwired: 2 in, 1 out]
            n94 = property on="Confirm 3rd Point" class="Bool"("DisabledEnum"=w169) -> ()  [unwired: 2 in, 2 out]
            n95 = property on="Cal Value 3" class="DigNum (strict)"(error in=w167, "Key Focus"=TRUE) -> ()  [unwired: 1 in, 2 out]
          }
          event "Confirm 3rd Point": Value Change {
            w173 = T10."Enabled" ("Disabled")
            w174 = T10."Disabled and Grayed Out" ("Disabled")
            n96 = event-data() -> ()  [unwired: 1 in, 1 out]
            n97 = property on="Reading Value 3" class="DigNum (strict)"("DisabledEnum"=w174) -> ()  [unwired: 2 in, 2 out]
            n98 = property on="Cal Value 3" class="DigNum (strict)"("DisabledEnum"=w174) -> ()  [unwired: 2 in, 2 out]
            n99 = property on="Confirm 3rd Point" class="Bool"("DisabledEnum"=w174) -> ()  [unwired: 2 in, 2 out]
            n100 = property on="Reading Value 4" class="DigNum (strict)"("DisabledEnum"=w173) -> ()  [unwired: 2 in, 2 out]
            n101 = property on="Cal Value 4" class="DigNum (strict)"("DisabledEnum"=w173) -> (error out=w172:errorcluster)  [unwired: 2 in, 1 out]
            n102 = property on="Confirm 4th Point" class="Bool"("DisabledEnum"=w173) -> ()  [unwired: 2 in, 2 out]
            n103 = property on="Cal Value 4" class="DigNum (strict)"(error in=w172, "Key Focus"=TRUE) -> ()  [unwired: 1 in, 2 out]
          }
          event "Confirm 4th Point": Value Change {
            w181 = T10."Enabled" ("Disabled")
            w182 = T10."Disabled and Grayed Out" ("Disabled")
            n104 = event-data() -> ()  [unwired: 1 in, 6 out]
            n105 = property on="Reading Value 4" class="DigNum (strict)"("DisabledEnum"=w182) -> ()  [unwired: 2 in, 2 out]
            n106 = property on="Cal Value 4" class="DigNum (strict)"("DisabledEnum"=w182) -> ()  [unwired: 2 in, 2 out]
            n107 = property on="Confirm 4th Point" class="Bool"("DisabledEnum"=w182) -> ()  [unwired: 2 in, 2 out]
            n108 = property on="Reading Value 5" class="DigNum (strict)"("DisabledEnum"=w181) -> ()  [unwired: 2 in, 2 out]
            n109 = property on="Cal Value 5" class="DigNum (strict)"("DisabledEnum"=w181) -> (error out=w180:errorcluster)  [unwired: 2 in, 1 out]
            n110 = property on="Confirm 5th Point" class="Bool"("DisabledEnum"=w181) -> ()  [unwired: 2 in, 2 out]
            n111 = property on="Cal Value 5" class="DigNum (strict)"(error in=w180, "Key Focus"=TRUE) -> ()  [unwired: 1 in, 2 out]
          }
          event "Confirm 5th Point": Value Change {
            n112 = event-data() -> ()  [unwired: 1 in, 6 out]
          }
          event "Cancel Cal": Value Change {
            n113 = event-data() -> ()  [unwired: 1 in, 1 out]
          }
          event "Verify Read": Value Change {
            n114 = event-data() -> ()  [unwired: 1 in, 1 out]
            n115 = case shown="True" "Verify Read" {
              tunnel: [FALSE ("Verify Read") FALSE ("Verify Read")] -> w193
              tunnel: w192 -> [_ _]
              tunnel: w192 -> [w197 w202]
              tunnel: [w197 w201] -> w191
              tunnel: [w195 string[] ["Calc Dev", "Cal Review"]] -> w188
              tunnel: w187 -> [w195 _]
              frame False {
              }
              frame True {
                n116 = local read "Row"() -> (w205:i32)
                n117 = local read "f(x)"() -> (w210:dbl)
                n118 = local read "Verify Table"() -> (w198:string[][])
                n119 = Number To Fractional String(number=w210) -> (F-format string=w204:string)  [unwired: 3 in]
                n120 = Replace Array Subset(array=w198, new element=w204, index (row)=w205, index (col)=1 ("disabled index (col)")) -> (w200:string[][])
                n121 = Increment(x=w205) -> (x+1=w209:i32)
                n122 = Bundle(w209, "disabled index (col)"=1) -> (w206:cluster{i32, "disabled index (col)":i32})  [unwired: 1 in]
                n123 = Bundle By Name(cluster=w202, "Verify Table"=w200) -> (w201:T9)
                n124 = property on="Verify Table" class="Tbl (strict)"("Key Focus"=TRUE, "EditPos"=w206, "Value"=w200) -> ()  [unwired: 2 in, 2 out]
              }
            }
            n125 = local write "Verify Read"(w193) -> ()
            n126 = Bundle By Name(cluster=w191, "Init Mean"=TRUE ("initialize")) -> (w190:T9)
          }
          event "Verify Edit": Value Change {
            n127 = event-data() -> ()  [unwired: 1 in, 1 out]
            n128 = case shown="False" "Verify Edit" {
              tunnel: w214 -> [w227 _]
              frame False {
                w228 = T10."Enabled" ("Disabled")
                n129 = Unbundle By Name(w227) -> ("Targets"=w223:T6, "Cal Targets Path"=w225:path, "Cal Unit"=w224:T1)
                n130 = local read "Verify Table"() -> (w226:string[][])
                n131 = Index Array(array=w226, index (col)=0 ("disabled index (col)")) -> (element=w217:string[])  [unwired: 1 in]
                n132 = Fract/Exp String To Number(string=w217) -> (number=w216:dbl[])  [unwired: 3 in, 1 out]
                n133 = Array To Cluster(array=w216) -> (cluster=w215:T14)
                n134 = case shown="\"mA\"" w224 {
                  tunnel: w223 -> [w233 w236 w239 w242 w245]
                  tunnel: [w232 w235 w238 w241 w244] -> w222
                  tunnel: w215 -> [w231 w234 w237 w240 w243]
                  frame "V", Default {
                    n135 = Bundle By Name(cluster=w233, "V Targets"=w231) -> (w232:T6)
                  }
                  frame "mA" {
                    n136 = Bundle By Name(cluster=w236, "mA Targets"=w234) -> (w235:T6)
                  }
                  frame "A" {
                    n137 = Bundle By Name(cluster=w239, "A Targets"=w237) -> (w238:T6)
                  }
                  frame "Hz" {
                    n138 = Bundle By Name(cluster=w242, "Hz Targets"=w240) -> (w241:T6)
                  }
                  frame "deg C" {
                    n139 = Bundle By Name(cluster=w245, "TC Targets"=w243) -> (w244:T6)
                  }
                }
                n140 = call <vilib>:"Open Config Data.vi"("configuration file path"=w225) -> ("error out"=w221:errorcluster, "refnum"=w220:T15)  [unwired: 8 in, 1 out]
                n141 = call <userlib>:"Write INI Cluster__ogtk.vi"("error in (no error)"=w221, "INI Fomatted Cluster"=w222, "refnum"=w220) -> ("error out"=w219:errorcluster, "dup refnum"=w218:T15)  [unwired: 7 in]
                n142 = property on="Hide Cal Values" class="Bool"("Visible"=TRUE) -> ()  [unwired: 2 in, 2 out]
                n143 = call <vilib>:"Close Config Data.vi"("error in (no error)"=w219, "refnum"=w218) -> ()  [unwired: 8 in, 2 out]
                n144 = property on="Verify Read" class="Bool (strict)"("DisabledEnum"=w228) -> ()  [unwired: 2 in, 2 out]
                n145 = property on="Auto" class="Bool (strict)"("DisabledEnum"=w228) -> ()  [unwired: 2 in, 2 out]
              }
              frame True {
                w246 = T10."Disabled and Grayed Out" ("Disabled")
                n146 = property on="Verify Read" class="Bool (strict)"("DisabledEnum"=w246) -> ()  [unwired: 2 in, 2 out]
                n147 = property on="Auto" class="Bool (strict)"("DisabledEnum"=w246) -> ()  [unwired: 2 in, 2 out]
                n148 = property on="Hide Cal Values" class="Bool"("Visible"=FALSE) -> ()  [unwired: 2 in, 2 out]
              }
            }
          }
          event "Save Cal": Value Change {
            n149 = event-data() -> ()  [unwired: 1 in, 1 out]
            n150 = property on="Cal Table" class="Tbl (strict)"("DisabledEnum"=T10."Enabled" ("Disabled")) -> ()  [unwired: 2 in, 2 out]
            n151 = property on="Verify Tab" class="TabCtl (strict)"("Visible"=FALSE) -> ()  [unwired: 2 in, 2 out]
          }
          event "Auto": Value Change {
            n152 = event-data() -> ()  [unwired: 1 in, 1 out]
            n153 = case shown="True" "Auto" {
              frame False {
              }
              frame True {
                n154 = local read "Row"() -> (w256:i32)
                n155 = Bundle("Row"=w256, "disabled index (col)"=1) -> (w257:cluster{"Row":i32, "disabled index (col)":i32})  [unwired: 1 in]
                n156 = property on="Verify Table" class="Tbl (strict)"("Key Focus"=TRUE, "EditPos"=w257) -> ()  [unwired: 2 in, 2 out]
              }
            }
            n157 = Bundle By Name(cluster=w254, "Auto"="Auto") -> (w253:T9)
          }
          event "Verify Table": Value Change {
            n158 = event-data() -> ()  [unwired: 1 in, 1 out]
            n159 = Bundle By Name(cluster=w263, "Verify Table"="Verify Table") -> (w262:T9)
          }
        }
      }
      frame "Init" {
        w265 = Units_Type_Def_(DAQ_Rack)."A" ("Cal Unit")
        # "#Change adding in new subVI for RIO"
        n160 = Unbundle By Name(w278) -> ("debug"=w276:bool, "App Dir"=w275:path)
        n161 = Select(t=path "C:/Users/zstreeter/Documents/Projects/Calibration Utility/Source", s=w276, f=w275) -> (s? t:f=w274:path)
        n162 = Build Path(base path=w274, name or relative path="App Config.ini") -> (appended path=w281:path)
        n163 = Build Path(base path=w274, name or relative path="Calibration UIs\\Durability Tank") -> (appended path=w272:path)
        n164 = call "Read App Config.vi"("App Config Path"=w281) -> ("Cal Files Path"=w285:path, "Registered Systems"=w269:T3[])  [unwired: 8 in, 1 out]
        n165 = Build Path(base path=w285, name or relative path="Durability Tank") -> (appended path=w280:path)
        n166 = Build Path(base path=w272, name or relative path="Cal Targets.ini") -> (appended path=w283:path)
        n167 = Create Folder(path (use dialog)=w280) -> (error out=w287:errorcluster)  [unwired: 2 in, 2 out]
        n168 = call <vilib>:"Clear Errors.vi"("error in (no error)"=w287) -> ("error out"=w279:errorcluster)  [unwired: 6 in]
        n169 = for {
          tunnel: [w294] -> w270 mode=indexing
          tunnel: w280 -> [w293]
          tunnel: w279 -> [w292]
          tunnel: w272 -> [w291]
          tunnel: string[] ["Durability Tank Cal Template.xls"] -> [w290] mode=indexing
          n170 = Build Path(base path=w293, name or relative path=w290) -> (appended path=w294:path)
          n171 = Build Path(base path=w291, name or relative path=w290) -> (appended path=w297:path)
          n172 = call <vilib>:"Check if File or Folder Exists.vi"("error in (no error)"=w292, "path"=w294) -> ("file or folder exists?"=w295:bool, "dup path"=w296:path)  [unwired: 7 in, 1 out]
          n173 = case shown="False" w295 {
            tunnel: w296 -> [w299 _]
            tunnel: w297 -> [w298 _]
            frame False {
              n174 = Copy(10:w299, 11:w298) -> ()  [unwired: 3 in, 3 out]
            }
            frame True {
            }
          }
        }
        n175 = Index Array(array=w270) -> (element=w264:path)  [unwired: 1 in]
        n176 = local write "Tank IP:"("" ("DAQ Rack")) -> ()
        n177 = call "Create Cal File Array (RIO).vi"() -> ("Cal Target Array"=w266:string[], "Cal Log OUT"=w267:string[][])  [unwired: 10 in]
        n178 = Bundle By Name(cluster=w278, "Registered Systems"=w269, "Cal Files Base Path"=w280, "Base Path"=w274, "Cal Targets Path"=w283, "Cal Template Path"=w264, "Default Cal Log"=w267, "Cal Target Array"=w266, "Cal Unit"=w265) -> (w289:T9)
        n179 = local write "Cal Unit"(w265) -> ()
      }
      frame "Unused Items" {
      }
      frame "Init Cal" {
        w303 = FALSE ("Auto")
        w309 = FALSE ("Verify Read")
        w310 = T10."Enabled" ("Disabled")
        w302 = T10."Disabled and Grayed Out" ("Disabled")
        n180 = Unbundle By Name(w314) -> ("Cal Log Header"=w305:string[])
        n181 = property on="Reading Value 1" class="DigNum (strict)"("DisabledEnum"=w302) -> ()  [unwired: 2 in, 2 out]
        n182 = property on="Cal Value 1" class="DigNum (strict)"("DisabledEnum"=w302) -> ()  [unwired: 2 in, 2 out]
        n183 = property on="Confirm 1st Point" class="Bool"("DisabledEnum"=w302) -> ()  [unwired: 2 in, 2 out]
        n184 = property on="Reading Value 2" class="DigNum (strict)"("DisabledEnum"=w302) -> ()  [unwired: 2 in, 2 out]
        n185 = property on="Cal Value 2" class="DigNum (strict)"("DisabledEnum"=w302) -> ()  [unwired: 2 in, 2 out]
        n186 = property on="Confirm 2nd Point" class="Bool"("DisabledEnum"=w302) -> ()  [unwired: 2 in, 2 out]
        n187 = property on="Reading Value 3" class="DigNum (strict)"("DisabledEnum"=w302) -> ()  [unwired: 2 in, 2 out]
        n188 = property on="Save Cal" class="Bool"("DisabledEnum"=w302) -> ()  [unwired: 2 in, 2 out]
        n189 = property on="Cancel Cal" class="Bool (strict)"("DisabledEnum"=w302) -> ()  [unwired: 2 in, 2 out]
        n190 = property on="Cal Table" class="Tbl (strict)"("Column Headers[]"=w305) -> ()  [unwired: 2 in, 2 out]
        n191 = property on="Cal Value 3" class="DigNum (strict)"("DisabledEnum"=w302) -> ()  [unwired: 2 in, 2 out]
        n192 = property on="Confirm 3rd Point" class="Bool"("DisabledEnum"=w302) -> ()  [unwired: 2 in, 2 out]
        n193 = property on="f(x)" class="DigNum (strict)"("DisabledEnum"=w302) -> ()  [unwired: 2 in, 2 out]
        n194 = property on="a0" class="DigNum (strict)"("DisabledEnum"=w302) -> ()  [unwired: 2 in, 2 out]
        n195 = property on="a1" class="DigNum (strict)"("DisabledEnum"=w302) -> ()  [unwired: 2 in, 2 out]
        n196 = property on="x" class="DigNum (strict)"("DisabledEnum"=w302) -> ()  [unwired: 2 in, 2 out]
        n197 = property on="a2" class="DigNum (strict)"("DisabledEnum"=w302) -> ()  [unwired: 2 in, 2 out]
        n198 = property on="a3" class="DigNum (strict)"("DisabledEnum"=w302) -> ()  [unwired: 2 in, 2 out]
        n199 = property on="a4" class="DigNum (strict)"("DisabledEnum"=w302) -> ()  [unwired: 2 in, 2 out]
        n200 = property on="Reading Value 4" class="DigNum (strict)"("DisabledEnum"=w302) -> ()  [unwired: 2 in, 2 out]
        n201 = property on="Cal Value 4" class="DigNum (strict)"("DisabledEnum"=w302) -> ()  [unwired: 2 in, 2 out]
        n202 = property on="Confirm 4th Point" class="Bool"("DisabledEnum"=w302) -> ()  [unwired: 2 in, 2 out]
        n203 = property on="Reading Value 5" class="DigNum (strict)"("DisabledEnum"=w302) -> ()  [unwired: 2 in, 2 out]
        n204 = property on="Cal Value 5" class="DigNum (strict)"("DisabledEnum"=w302) -> ()  [unwired: 2 in, 2 out]
        n205 = property on="Confirm 5th Point" class="Bool"("DisabledEnum"=w302) -> ()  [unwired: 2 in, 2 out]
        n206 = property on="Verify Read" class="Bool (strict)"("DisabledEnum"=w310) -> ()  [unwired: 2 in, 2 out]
        n207 = property on="Cal Table" class="Tbl (strict)"("DisabledEnum"=w310) -> ()  [unwired: 2 in, 2 out]
        n208 = local write "Auto"(w309) -> ()
        n209 = local write "Verify Edit"(w309) -> ()
        n210 = property on="Verify Tab" class="TabCtl (strict)"("Visible"=FALSE) -> ()  [unwired: 2 in, 2 out]
        n211 = property on="Hide Cal Values" class="Bool"("Visible"=TRUE) -> ()  [unwired: 2 in, 2 out]
        n212 = local write "Verify Read"(w309) -> ()
        n213 = Bundle By Name(cluster=w314, "Auto"=w303, "Verification"=w303) -> (w313:T9)
        n214 = Insert Into Array(array=w307, index=0, new element=string[] ["Clear Dev Data", "Update Dev Tables", "Load Template"]) -> (w304:string[])
      }
      frame "Check for RIO" {
        n215 = Unbundle By Name(w316) -> ("Desired System.Serial Number"=w315:string, "Verification"=w320:bool)
        n216 = call "Find Network Systems.vi"() -> ("Serial Number"=w318:string)  [unwired: 10 in, 1 out]
        n217 = Equal?(x=w318, y=w315) -> (x = y?=w317:bool)
        n218 = case shown="True" w317 {
          tunnel: w320 -> [w324 _]
          tunnel: [w325 string[] []] -> w319
          frame True {
            # "Desired system found."
            n219 = case shown="False" w324 {
              tunnel: [string[] ["Set Relay", "Load Targets", "Calculate Coeffs"] string[] ["Set Relay", "Load Targets", "Start Cal"]] -> w325
              frame True {
              }
              frame False {
              }
            }
          }
          frame False {
            w329 = T10."Enabled" ("Disabled")
            # "Couldn't find desired system."
            n220 = property on="Start Cal" class="Bool"("DisabledEnum"=w329) -> ()  [unwired: 2 in, 2 out]
            n221 = property on="Header" class="Bool"("DisabledEnum"=w329) -> ()  [unwired: 2 in, 2 out]
            n222 = One Button Dialog(message="Couldn't connect to desired DAQ hardware.") -> ()  [unwired: 1 in, 1 out]
          }
        }
        n223 = Insert Into Array(array=w322, index=0, new element=w319) -> (w321:string[])
      }
      frame "Adjust Channels" {
        n224 = Unbundle By Name(w344) -> ("Desired System.ID"=w334:string, "Desired System.System Type"=w345:T4, "Channel to Cal"=w340:T2, "Cal Unit"=w336:T1)
        n225 = property on="Channel to Cal" class="Enum (strict)"() -> ("NumItems"=w332:u32)  [unwired: 2 in, 2 out]
        n226 = property on="Cal Unit" class="Enum (strict)"() -> ("Strings []"=w341:string[])  [unwired: 2 in, 2 out]
        n227 = Decimal String To Number(string=w334) -> (number=w333:i32)  [unwired: 2 in, 1 out]
        n228 = case shown="\"RIO\"" w345 {
          tunnel: [w361 Rack_Version_Type_Def."RIO" Rack_Version_Type_Def."Cart"] -> w342
          tunnel: w332 -> [w356 w474 w498]
          tunnel: [w360 w478 w502] -> w331
          tunnel: w341 -> [w359 w476 w500]
          tunnel: [w358 w475 w499] -> w337
          tunnel: w340 -> [w357 _ _]
          tunnel: w333 -> [w355 _ _]
          frame "DAQ Rack", Default {
            n229 = disable-structure shown="Enabled" {
              disable-tunnel: [w368 _] -> w361
              disable-tunnel: [w367 _] -> w360
              disable-tunnel: w359 -> [w366 _]
              disable-tunnel: [w365 _] -> w358
              disable-tunnel: w357 -> [w364 _]
              disable-tunnel: w356 -> [w363 _]
              disable-tunnel: w355 -> [w362 _]
              frame Disabled {
                n230 = case shown="1..4, Default" w362 {
                  tunnel: [Rack_Version_Type_Def."Volts & TC" Rack_Version_Type_Def."Volts" Rack_Version_Type_Def."Volts & Current"] -> w368
                  tunnel: [w374 w409 w434] -> w367
                  tunnel: w366 -> [w372 w411 w437]
                  tunnel: [w371 w408 w433] -> w365
                  tunnel: w364 -> [w370 _ w436]
                  tunnel: w363 -> [w369 w412 w438]
                  frame 1..4, Default {
                    n231 = for {
                      N: w369 -> [_]
                      shift-right: [w402] -> w374
                      shift-left: i32[] [] ("Disabled Items []") -> [w403]
                      i -> [w401]
                      n232 = case shown="32..47" w401 {
                        tunnel: w403 -> [w404 w407]
                        tunnel: [w404 w405] -> w402
                        tunnel: w401 -> [_ w406]
                        frame 0..31, 48..63, Default {
                        }
                        frame 32..47 {
                          n233 = Build Array (concatenate)(w407, w406) -> (w405:i32[])
                        }
                      }
                    }
                    n234 = for {
                      tunnel: w372 -> [w381] mode=indexing
                      shift-right: [w379] -> w371
                      shift-left: i32[] [] ("Disabled Items []") -> [w380]
                      tunnel: w370 -> [w377]
                      i -> [w378]
                      n235 = case shown="\"deg C\"" w381 {
                        tunnel: w380 -> [w385 w392 w400]
                        tunnel: [w383 w391 w398] -> w379
                        tunnel: w378 -> [w384 w390 w399]
                        tunnel: w377 -> [w382 w393 _]
                        frame "Hz", "V", Default {
                          n236 = case shown="\"AI-00 Pos 1 Pump Current\"..\"AI-31 Pos 4 Flow\", Default" w382 {
                            tunnel: [w386 w387] -> w383
                            tunnel: w385 -> [w386 w389]
                            tunnel: w384 -> [_ w388]
                            frame "AI-00 Pos 1 Pump Current".."AI-31 Pos 4 Flow", Default {
                            }
                            frame "AI-00 Pos 1 Pump Current", "AI-01 Pos 2 Pump Current" {
                              n237 = Build Array (concatenate)(w389, w388) -> (w387:i32[])
                            }
                          }
                        }
                        frame "deg C" {
                          n238 = case shown="\"TC-00\"..\"TC-15\"" w393 {
                            tunnel: [w394 w397] -> w391
                            tunnel: w392 -> [w396 w397]
                            tunnel: w390 -> [w395 _]
                            frame "AI-00 Pos 1 Pump Current".."AI-31 Pos 4 Flow", Default {
                              n239 = Build Array (concatenate)(w396, w395) -> (w394:i32[])
                            }
                            frame "AI-00 Pos 1 Pump Current", "AI-01 Pos 2 Pump Current" {
                            }
                          }
                        }
                        frame "A", "mA" {
                          n240 = Build Array (concatenate)(w400, w399) -> (w398:i32[])
                        }
                      }
                    }
                  }
                  frame 5..8 {
                    n241 = for {
                      N: w412 -> [_]
                      shift-right: [w424] -> w409
                      shift-left: i32[] [] ("Disabled Items []") -> [w425]
                      i -> [w423]
                      n242 = case shown="48..63" w423 {
                        tunnel: w425 -> [w426 w429 w432]
                        tunnel: [w426 w427 w430] -> w424
                        tunnel: w423 -> [_ w428 w431]
                        frame 0..31, Default {
                        }
                        frame 32..47 {
                          n243 = Build Array (concatenate)(w429, w428) -> (w427:i32[])
                        }
                        frame 48..63 {
                          n244 = Build Array (concatenate)(w432, w431) -> (w430:i32[])
                        }
                      }
                    }
                    n245 = for {
                      tunnel: w411 -> [w418] mode=indexing
                      shift-right: [w416] -> w408
                      shift-left: i32[] [] ("Disabled Items []") -> [w417]
                      i -> [w415]
                      n246 = case shown="\"Hz\", \"V\", Default" w418 {
                        tunnel: w417 -> [w419 w422]
                        tunnel: [w419 w420] -> w416
                        tunnel: w415 -> [_ w421]
                        frame "Hz", "V", Default {
                        }
                        frame "A", "deg C", "mA" {
                          n247 = Build Array (concatenate)(w422, w421) -> (w420:i32[])
                        }
                      }
                    }
                  }
                  frame 2000..2999 {
                    n248 = for {
                      N: w438 -> [_]
                      shift-right: [w466] -> w434
                      shift-left: i32[] [] ("Disabled Items []") -> [w467]
                      i -> [w465]
                      n249 = case shown="48..63" w465 {
                        tunnel: w467 -> [w468 w469 w472]
                        tunnel: [w468 w469 w470] -> w466
                        tunnel: w465 -> [_ _ w471]
                        frame 0..31, Default {
                        }
                        frame 32..47 {
                        }
                        frame 48..63 {
                          n250 = Build Array (concatenate)(w472, w471) -> (w470:i32[])
                        }
                      }
                    }
                    n251 = for {
                      tunnel: w437 -> [w445] mode=indexing
                      shift-right: [w443] -> w433
                      shift-left: i32[] [] ("Disabled Items []") -> [w444]
                      tunnel: w436 -> [w441]
                      i -> [w442]
                      n252 = case shown="\"Hz\", \"V\", Default" w445 {
                        tunnel: w444 -> [w449 w457 w464]
                        tunnel: [w446 w454 w462] -> w443
                        tunnel: w442 -> [w447 w456 w463]
                        tunnel: w441 -> [w448 w455 _]
                        frame "Hz", "V", Default {
                          n253 = case shown="Default, \"AI-32\"..\"AI-47\"" w448 {
                            tunnel: [w450 w453] -> w446
                            tunnel: w449 -> [w452 w453]
                            tunnel: w447 -> [w451 _]
                            frame "AI-00 Pos 1 Pump Current", "AI-01 Pos 2 Pump Current", Default {
                              n254 = Build Array (concatenate)(w452, w451) -> (w450:i32[])
                            }
                            frame "AI-00 Pos 1 Pump Current".."AI-31 Pos 4 Flow" {
                            }
                          }
                        }
                        frame "A", "mA" {
                          n255 = case shown="\"AI-00 Pos 1 Pump Current\"..\"AI-31 Pos 4 Flow\"" w455 {
                            tunnel: [w458 w459] -> w454
                            tunnel: w457 -> [w458 w461]
                            tunnel: w456 -> [_ w460]
                            frame "AI-00 Pos 1 Pump Current", "AI-01 Pos 2 Pump Current", Default {
                            }
                            frame "AI-00 Pos 1 Pump Current".."AI-31 Pos 4 Flow" {
                              n256 = Build Array (concatenate)(w461, w460) -> (w459:i32[])
                            }
                          }
                        }
                        frame "deg C" {
                          n257 = Build Array (concatenate)(w464, w463) -> (w462:i32[])
                        }
                      }
                    }
                  }
                }
              }
              frame Enabled {
              }
            }
          }
          frame "RIO" {
            # "#Change 1st case from 00..31 to 00..37\n                2nd case from 32..47 to 38..47"
            # "#Change Added \"A\" to RIO selection"
            n258 = for {
              N: w474 -> [_]
              shift-right: [w489] -> w478
              shift-left: i32[] [] ("Disabled Items []") -> [w490]
              i -> [w488]
              n259 = case shown="0..37, Default" w488 {
                tunnel: w490 -> [w491 w494 w497]
                tunnel: [w491 w492 w495] -> w489
                tunnel: w488 -> [_ w493 w496]
                frame 0..37, Default {
                }
                frame 38..47 {
                  n260 = Build Array (concatenate)(w494, w493) -> (w492:i32[])
                }
                frame 48..63 {
                  n261 = Build Array (concatenate)(w497, w496) -> (w495:i32[])
                }
              }
            }
            n262 = for {
              tunnel: w476 -> [w483] mode=indexing
              shift-right: [w481] -> w475
              shift-left: i32[] [] ("Disabled Items []") -> [w482]
              i -> [w480]
              n263 = case shown="\"Hz\", \"deg C\", \"mA\"" w483 {
                tunnel: w482 -> [w484 w487]
                tunnel: [w484 w485] -> w481
                tunnel: w480 -> [_ w486]
                frame "A", "V", Default {
                }
                frame "Hz", "deg C", "mA" {
                  n264 = Build Array (concatenate)(w487, w486) -> (w485:i32[])
                }
              }
            }
          }
          frame "DAQ Cart" {
            n265 = for {
              N: w498 -> [_]
              shift-right: [w514] -> w502
              shift-left: i32[] [] ("Disabled Items []") -> [w515]
              i -> [w513]
              n266 = case shown="48..63" w513 {
                tunnel: w515 -> [w516 w519 w522]
                tunnel: [w516 w517 w520] -> w514
                tunnel: w513 -> [_ w518 w521]
                frame 0..31, Default {
                }
                frame 32..47 {
                  n267 = Build Array (concatenate)(w519, w518) -> (w517:i32[])
                }
                frame 48..63 {
                  n268 = Build Array (concatenate)(w522, w521) -> (w520:i32[])
                }
              }
            }
            n269 = for {
              tunnel: w500 -> [w508] mode=indexing
              shift-right: [w506] -> w499
              shift-left: i32[] [] ("Disabled Items []") -> [w507]
              i -> [w505]
              n270 = case shown="\"A\", \"deg C\", \"mA\"" w508 {
                tunnel: w507 -> [w509 w512]
                tunnel: [w509 w510] -> w506
                tunnel: w505 -> [_ w511]
                frame "Hz", "V", Default {
                }
                frame "A", "deg C", "mA" {
                  n271 = Build Array (concatenate)(w512, w511) -> (w510:i32[])
                }
              }
            }
          }
        }
        n272 = property on="Channel to Cal" class="Enum (strict)"("Disabled Items []"=w331) -> ()  [unwired: 2 in, 2 out]
        n273 = property on="Cal Unit" class="Enum (strict)"("Disabled Items []"=w337) -> ()  [unwired: 2 in, 2 out]
        n274 = Search 1D Array(1D array=w337, element=w336) -> (index of element=w339:i32)  [unwired: 1 in]
        n275 = Greater Or Equal To 0?(x=w339) -> (x >= 0?=w338:bool)
        n276 = case shown="True" w338 {
          tunnel: [w347 w348] -> w335
          tunnel: w336 -> [w347 _]
          tunnel: w337 -> [_ w350]
          frame False {
          }
          frame True {
            n277 = for {
              N: 5 -> [_]
              tunnel: w350 -> [w354]
              tunnel: [w351] -> w348
              i -> [w351]
              stop <- w352 stop-if-true
              n278 = Search 1D Array(1D array=w354, element=w351) -> (index of element=w353:i32)  [unwired: 1 in]
              n279 = Less Than 0?(x=w353) -> (x < 0?=w352:bool)
            }
            n280 = local write "Cal Unit"(w348) -> ()
          }
        }
        n281 = Bundle By Name(cluster=w344, "Rack Version"=w342, "Cal Unit"=w335) -> (w343:T9)
      }
      frame "Button State" {
        n282 = Unbundle By Name(w525) -> ("Cal Unit"=w524:T1)
        n283 = case shown="Default" w524 {
          tunnel: [T10."Enabled" ("Disabled") T10."Disabled and Grayed Out" ("Disabled")] -> w523
          frame Default {
          }
          frame "deg C" {
          }
        }
        n284 = property on="Start Cal" class="Bool"("DisabledEnum"=w523) -> ()  [unwired: 2 in, 2 out]
      }
      frame "Clear Dev Data" {
        n285 = Bundle By Name(cluster=w531, "Verify Table"=string[][] [["", "", "", "", ""], ["", "", "", "", ""], ["", "", "", "", ""], ["", "", "", "", ""], ["", "", "", "", ""], ["", "", "", "", ""], ["", "", "", "", ""], ["", "", "", "", ""], ["", "", "", "", ""], ["", "", "", "", ""]]) -> (w530:T9)
      }
      frame "Update Dev Tables" {
        n286 = Unbundle By Name(w534) -> ("Verify Table"=w533:string[][])
        n287 = local write "Verify Table"(w533) -> ()
      }
      frame "Load Template" {
        n288 = Unbundle By Name(w537) -> ("Cal Template Path"=w542:path)
        n289 = call <vilib>:"Check if File or Folder Exists.vi"("path"=w542) -> ("file or folder exists?"=w541:bool)  [unwired: 8 in, 2 out]
        n290 = case shown="True" w541 {
          tunnel: [string[] [] string[] []] -> w540
          tunnel: w542 -> [w549 w552]
          tunnel: [FALSE ("Visible") FALSE ("Visible")] -> w543
          tunnel: [w546 w554] -> w544
          tunnel: [w546 w554] -> w545
          frame False {
            w546 = T10."Disabled and Grayed Out" ("Disabled")
            n291 = Format Into String(format string="Can't find cal spreadsheet template!\n\nShould have been here:  \"%s\"" ("message"), w549) -> (resulting string=w548:string)  [unwired: 2 in, 1 out]
            n292 = One Button Dialog(message=w548) -> ()  [unwired: 1 in, 1 out]
          }
          frame True {
            w554 = T10."Enabled" ("Disabled")
            n293 = call "Read Write Header.vi"("Cal Template Path"=w552, "Write (F)"=FALSE) -> ("Header Table 1"=w560:string[][], "Header Table 2"=w559:string[][], "Sys Cal Table"=w556:string[][], "Cal Standards Table"=w555:string[][], "Header Comments"=w557:string[][])  [unwired: 13 in]
            n294 = local write "Header Comments"(w557) -> ()
            n295 = local write "Cal Standards Table"(w555) -> ()
            n296 = local write "Header Table 1"(w560) -> ()
            n297 = local write "Header Table 2"(w559) -> ()
            n298 = local write "Sys Cal Table"(w556) -> ()
          }
        }
        n299 = property on="Load Indicator Tab" class="TabCtl (strict)"("Visible"=w543) -> ()  [unwired: 2 in, 2 out]
        n300 = property on="Header OK" class="Bool"("DisabledEnum"=w544) -> ()  [unwired: 2 in, 2 out]
        n301 = property on="Header Cancel" class="Bool"("DisabledEnum"=w545) -> ()  [unwired: 2 in, 2 out]
        n302 = Insert Into Array(array=w539, index=0, new element=w540) -> (w538:string[])
      }
      frame "Create Spreadsheet" {
        n303 = Unbundle By Name(w572) -> ("Rack Version"=w567:T5, "DAQ Rack"=w563:string, "Cal Files Base Path"=w574:path)
        n304 = Format Into String(format string="%s.xls", w563) -> (resulting string=w562:string)  [unwired: 2 in, 1 out]
        n305 = case shown="\"RIO\"" w567 {
          tunnel: ["DAQ Rack Cal Template.xls" ("name or relative path") "DAQ Cart Cal Template.xls" ("name or relative path") "Durability Tank Cal Template.xls" ("name or relative path")] -> w566
          frame Default {
          }
          frame "Cart" {
          }
          frame "RIO" {
          }
        }
        n306 = Build Path(base path=w574, name or relative path=w562) -> (appended path=w576:path)
        n307 = Empty String/Path?(string/path=w563) -> (empty?=w565:bool)
        n308 = Not A Number/Path/Refnum?(number/path/refnum=w576) -> (NaN/Path/Refnum?=w577:bool)
        n309 = Or(x=w577, y=w565) -> (x .or. y?=w578:bool)
        n310 = Build Path(base path=w574, name or relative path=w566) -> (appended path=w575:path)
        n311 = case shown="False" w578 {
          tunnel: [string[] ["Save Header"] string[] []] -> w573
          tunnel: w576 -> [w583 _]
          tunnel: w575 -> [w584 _]
          frame False {
            n312 = call <vilib>:"Check if File or Folder Exists.vi"("path"=w583) -> ("file or folder exists?"=w586:bool)  [unwired: 8 in, 2 out]
            n313 = case shown="True" w586 {
              tunnel: [FALSE ("T button?") w590] -> w585
              frame False {
              }
              frame True {
                n314 = Two Button Dialog(message="Cal file already exists.  How do you want to proceed?\n\n\"Use Existing\" will continue with existing file and data.  \"Overwrite\" will destroy all data and start with fresh template", 1:"Overwrite" ("F button name (\"Cancel\")"), 2:"Use Existing" ("T button name (\"OK\")")) -> (T button?=w590:bool)
              }
            }
            n315 = case shown="False" w585 {
              tunnel: w583 -> [w594 _]
              tunnel: w584 -> [w593 _]
              frame False {
                n316 = Copy(9:TRUE ("overwrite (F)"), 10:w594, 11:w593) -> ()  [unwired: 2 in, 3 out]
              }
              frame True {
              }
            }
          }
          frame True {
            w595 = T10."Enabled" ("Disabled")
            n317 = property on="Load Indicator Tab" class="TabCtl (strict)"("Visible"=FALSE) -> ()  [unwired: 2 in, 2 out]
            n318 = property on="Header OK" class="Bool"("DisabledEnum"=w595) -> ()  [unwired: 2 in, 2 out]
            n319 = property on="Header Cancel" class="Bool"("DisabledEnum"=w595) -> ()  [unwired: 2 in, 2 out]
            n320 = One Button Dialog(message="\"Manufacturer Serial #\" is blank or contains invalid characters.") -> ()  [unwired: 1 in, 1 out]
          }
        }
        n321 = Bundle By Name(cluster=w572, "Cal Spreadsheet Path"=w576) -> (w571:T9)
        n322 = Insert Into Array(array=w569, index=0, new element=w573) -> (w570:string[])
      }
      frame "Save Header" {
        n323 = Unbundle By Name(w607) -> ("Cal Spreadsheet Path"=w610:path, "Cal Template Path"=w611:path)
        n324 = Build Array(w610, w611) -> (w612:path[])
        n325 = for {
          tunnel: "Header Table 2" -> [w620]
          tunnel: "Sys Cal Table" -> [w619]
          tunnel: "Cal Standards Table" -> [w618]
          tunnel: "Header Comments" -> [w617]
          tunnel: [w616] -> w609
          tunnel: "Header Table 1" -> [w614]
          tunnel: w612 -> [w613] mode=indexing
          n326 = call "Read Write Header.vi"("Header Table 1 IN"=w614, "Header Table 2 IN"=w620, "Sys Cal Table IN"=w619, "Cal Standards Table IN"=w618, "Header Comments IN"=w617, "Cal Template Path"=w613, "Write (F)"=TRUE) -> ("Header Table 1"=w616:string[][])  [unwired: 8 in, 4 out]
        }
        n327 = flat-sequence {
          tunnel: w609 -> [_]
          frame #0 {
            w621 = T10."Enabled" ("Disabled")
            w622 = FALSE ("Visible")
            n328 = property on="View Spreadsheet" class="Bool"("DisabledEnum"=w621) -> ()  [unwired: 2 in, 2 out]
            n329 = property on="Main Tab" class="TabCtl (strict)"("DisabledEnum"=w621) -> ()  [unwired: 2 in, 2 out]
            n330 = property on="Tank IP:" class="Str"("DisabledEnum"=w621) -> ()  [unwired: 2 in, 2 out]
            n331 = property on="Channel to Cal" class="Enum (strict)"("DisabledEnum"=w621) -> ()  [unwired: 2 in, 2 out]
            n332 = property on="Cal Unit" class="Enum (strict)"("DisabledEnum"=w621) -> ()  [unwired: 2 in, 2 out]
            n333 = property on="Start Cal" class="Bool"("DisabledEnum"=w621) -> ()  [unwired: 2 in, 2 out]
            n334 = property on="Start Verification" class="Bool"("DisabledEnum"=w621) -> ()  [unwired: 2 in, 2 out]
            n335 = property on="Load Indicator Tab" class="TabCtl (strict)"("Visible"=w622) -> ()  [unwired: 2 in, 2 out]
            n336 = property on="Header Tab" class="TabCtl (strict)"("Visible"=w622) -> ()  [unwired: 2 in, 2 out]
          }
        }
        n337 = Insert Into Array(array=w605, index=0, new element=string[] []) -> (w606:string[])
      }
      frame "Create Cal File" {
        n338 = Unbundle By Name(w626) -> ("Cal Files Base Path"=w628:path, "Cal Log Header"=w631:string[], "Default Cal Log"=w630:string[][])
        n339 = local read "Tank IP:"() -> (w623:string)
        n340 = Build Array (concatenate)(w631, w630) -> (w629:string[][])
        n341 = case shown="Default" w623 {
          tunnel: w629 -> [w640 _]
          tunnel: w628 -> [w639 _]
          tunnel: w623 -> [w637 _]
          tunnel: [w638 path "" ("dup path")] -> w624
          frame Default {
            n342 = Format Into String(format string="%s.cal", w637) -> (resulting string=w635:string)  [unwired: 2 in, 1 out]
            n343 = Build Path(base path=w639, name or relative path=w635) -> (appended path=w643:path)
            n344 = call <vilib>:"Check if File or Folder Exists.vi"("path"=w643) -> ("file or folder exists?"=w642:bool, "dup path"=w641:path)  [unwired: 8 in, 1 out]
            n345 = case shown="False" w642 {
              tunnel: w641 -> [w647 w648]
              tunnel: w640 -> [w646 _]
              tunnel: [w644 w648] -> w638
              frame False {
                n346 = call-poly <vilib>:"Write To Spreadsheet File.vi"("delimiter (\\t)"="," ("delimiter (\\t)"), "2D data"=w646, "file path (dialog if empty)"=w647) -> ("new file path (Not A Path if cancelled)"=w644:path)  [unwired: 5 in]
              }
              frame True {
              }
            }
          }
          frame "" {
          }
        }
        n347 = Insert Into Array(array=w632, index=0, new element=string[] ["Load Cal File"]) -> (w633:string[])
        n348 = Bundle By Name(cluster=w626, "Cal File Path"=w624) -> (w625:T9)
      }
      frame "Load Cal File" {
        n349 = Unbundle By Name(w654) -> ("Default Cal Log"=w650:string[][], "Cal File Path"=w651:path)
        n350 = Empty String/Path?(string/path=w651) -> (empty?=w652:bool)
        n351 = case shown="False" w652 {
          tunnel: w651 -> [w661 _]
          tunnel: [w665 w702] -> w658
          tunnel: [w663 string[] []] -> w655
          tunnel: w654 -> [w662 w702]
          tunnel: w650 -> [w659 _]
          frame False {
            n352 = call <vilib>:"Check if File or Folder Exists.vi"("path"=w661) -> ("file or folder exists?"=w664:bool, "dup path"=w660:path)  [unwired: 8 in, 1 out]
            n353 = case shown="True" w664 {
              tunnel: w660 -> [_ w696]
              tunnel: w662 -> [w666 w693]
              tunnel: [w666 w692] -> w665
              tunnel: [string[] ["Create Cal File"] string[] []] -> w663
              tunnel: w659 -> [_ w689]
              frame False {
              }
              frame True {
                w688 = 0 ("index (row)")
                n354 = call-poly <vilib>:"Read From Spreadsheet File.vi"("delimiter (\\t)"="," ("delimiter (\\t)"), "file path (dialog if empty)"=w696) -> ("all rows"=w695:string[][])  [unwired: 5 in, 4 out]
                n355 = Delete From Array(array=w695, index (row)=0) -> (array with subset deleted=w684:string[][])  [unwired: 2 in, 1 out]
                n356 = Index Array(array=w684, index (col)=0 ("disabled index (col)")) -> (element=w686:string[])  [unwired: 1 in]
                n357 = Search 1D Array(1D array=w686, element="") -> (index of element=w682:i32)  [unwired: 1 in]
                n358 = Delete From Array(array=w684, index (row)=w682) -> (array with subset deleted=w683:string[][])  [unwired: 2 in, 1 out]
                n359 = Replace Array Subset(array=w689, new element=w683, index (row)=w688, index (col)=w688) -> (w676:string[][])
                n360 = Index Array(array=w676, index (col)=1 ("disabled index (col)")) -> (element=w669:string[])  [unwired: 1 in]
                n361 = for {
                  tunnel: w669 -> [w698] mode=indexing
                  tunnel: [w697] -> w668 mode=indexing
                  n362 = case shown="\"V\", Default" w698 {
                    tunnel: ["V" "A"] -> w697
                    frame "V", Default {
                    }
                    frame "A" {
                    }
                  }
                }
                n363 = Array To Spreadsheet String(array=w668, 3:"%s" ("format string")) -> (spreadsheet string=w680:string)  [unwired: 1 in]
                n364 = Search and Replace String(replace all?=TRUE ("replace all? (F)"), input string=w680, search string="degC", replace string="deg C" ("search string")) -> (result string=w673:string)  [unwired: 4 in, 3 out]
                n365 = Spreadsheet String To Array(format string="%s", spreadsheet string=w673, array type (2D Dbl)=w668) -> (array=w672:string[])  [unwired: 1 in]
                n366 = Replace Array Subset(array=w676, new element=w672, index (col)=1 ("disabled index (col)")) -> (w675:string[][])  [unwired: 1 in]
                n367 = Bundle By Name(cluster=w693, "Cal Log"=w675) -> (w692:T9)
                n368 = property on="Cal Table" class="Tbl (strict)"("Value"=w675) -> ()  [unwired: 2 in, 2 out]
              }
            }
          }
          frame True {
          }
        }
        n369 = Insert Into Array(array=w656, index=0, new element=w655) -> (w657:string[])
      }
      frame "Load Targets" {
        w717 = 0 ("length")
        w711 = T10."Disabled and Grayed Out" ("Disabled")
        # "#Change In \"A\" selection added selection of \"RIO\" that links 25A Targets and Setpoints"
        n370 = Unbundle By Name(w721) -> ("Cal Targets Path"=w728:path, "Targets"=w723:T6, "Cal Target Array"=w706:string[], "Channel to Cal"=w705:T2, "Verify Table"=w734:string[][])
        n371 = property on="Cancel Cal" class="Bool (strict)"("DisabledEnum"=T10."Enabled" ("Disabled")) -> ()  [unwired: 2 in, 2 out]
        n372 = property on="Cal Table" class="Tbl (strict)"("Active Cell"=T11 {"Row"=-2, "Column"=-2} ("Active Cell:Active Cell"), "Cell BG Color"=u32 16448250) -> ()  [unwired: 2 in, 2 out]
        n373 = call <vilib>:"Open Config Data.vi"("configuration file path"=w728) -> ("error out"=w726:errorcluster, "refnum"=w727:T15)  [unwired: 8 in, 1 out]
        n374 = property on="Tank IP:" class="Str"("DisabledEnum"=w711) -> ()  [unwired: 2 in, 2 out]
        n375 = property on="Channel to Cal" class="Enum (strict)"("DisabledEnum"=w711) -> ()  [unwired: 2 in, 2 out]
        n376 = property on="Cal Unit" class="Enum (strict)"("DisabledEnum"=w711) -> ()  [unwired: 2 in, 2 out]
        n377 = property on="Start Cal" class="Bool"("DisabledEnum"=w711) -> ()  [unwired: 2 in, 2 out]
        n378 = property on="Start Verification" class="Bool"("DisabledEnum"=w711) -> ()  [unwired: 2 in, 2 out]
        n379 = call <userlib>:"Read INI Cluster__ogtk.vi"("error in (no error)"=w726, "INI Fomatted Cluster Type"=w723, "refnum"=w727) -> ("error out"=w724:errorcluster, "INI Fomatted Cluster"=w722:variant, "dup refnum"=w725:T15)  [unwired: 4 in, 2 out]
        n380 = Index Array(array=w706, index=w705) -> (element=w710:string)
        n381 = call <vilib>:"Close Config Data.vi"("error in (no error)"=w724, "refnum"=w725) -> ()  [unwired: 8 in, 2 out]
        n382 = Variant To Data(type=w723, Variant=w722) -> (data=w709:T6)  [unwired: 1 in, 1 out]
        n383 = case shown="\"CT\"" w710 {
          tunnel: w709 -> [w742 w745 w748 w751 w754 w757]
          tunnel: [w740 w743 w746 w749 w752 w755] -> w707
          tunnel: [w741 w744 w747 w750 w753 w756] -> w708
          frame "V", Default {
            n384 = Unbundle By Name(w742) -> ("V Targets"=w741:T7, "V Setpoints"=w740:T8)
          }
          frame "A" {
            n385 = Unbundle By Name(w745) -> ("A Targets"=w744:T7, "A Setpoints"=w743:T8)
          }
          frame "DegC" {
            n386 = Unbundle By Name(w748) -> ("DegC Targets"=w747:T7, "DegC Setpoints"=w746:T8)
          }
          frame "kPa" {
            n387 = Unbundle By Name(w751) -> ("kPa Targets"=w750:T7, "kPa Setpoints"=w749:T8)
          }
          frame "LpH" {
            n388 = Unbundle By Name(w754) -> ("LpH Targets"=w753:T7, "LpH Setpoints"=w752:T8)
          }
          frame "CT" {
            n389 = Unbundle By Name(w757) -> ("CT Targets"=w756:T7, "CT Setpoints"=w755:T8)
          }
        }
        n390 = Cluster To Array(cluster=w708) -> (array=w718:dbl[])
        n391 = Cluster To Array(cluster=w707) -> (array=w719:dbl[])
        n392 = Delete From Array(array=w718, length=w717, index=w717) -> (deleted portion=w713:dbl[], array with subset deleted=w716:dbl[])
        n393 = call-poly <userlib>:"Remove Duplicates from 1D Array__ogtk.vi"("Input Array"=w716) -> ("Output Array"=w715:dbl[])  [unwired: 1 out]
        n394 = Build Array (concatenate)(w713, w715) -> (w714:dbl[])
        n395 = Number To Fractional String(number=w714, precision (6)=i16 3) -> (F-format string=w720:string[])  [unwired: 2 in]
        n396 = Index Array(array=w719) -> (element #1=w731:dbl, element #2=w730:dbl, element #3=w729:dbl, element #4=w704:dbl, element #5=w703:dbl)  [unwired: 5 in]
        n397 = Replace Array Subset(array=w734, new element=w720, index (col)=0 ("disabled index (col)")) -> (w732:string[][])  [unwired: 1 in]
        n398 = local write "Cal Value 1"(w731) -> ()
        n399 = local write "Cal Value 2"(w730) -> ()
        n400 = local write "Cal Value 3"(w729) -> ()
        n401 = local write "Cal Value 4"(w704) -> ()
        n402 = local write "Cal Value 5"(w703) -> ()
        n403 = Bundle By Name(cluster=w721, "Targets"=w709, "Verify Table"=w732) -> (w735:T9)
        n404 = property on="Verify Table" class="Tbl (strict)"("Value"=w732) -> ()  [unwired: 2 in, 2 out]
      }
      frame "Set Relay" {
        n405 = Unbundle By Name(w761) -> ("Selected Chassis"=w759:tag, "Channel to Cal"=w758:T2, "Cal Unit"=w760:T1)
        n406 = case shown="\"mA\"" w760 {
          tunnel: w759 -> [_ w770]
          tunnel: w758 -> [_ w768]
          frame Default {
          }
          frame "mA" {
            # "Turn on parasitic relay."
            n407 = property class="DAQmx Device"("Active Device"=w770) -> ("Chassis.ModuleDevNames"=w772:tag[])  [unwired: 2 in, 2 out]
            n408 = Subtract(x=w768, y=Channel_Type_Def_(RIO)."AI-32 Pos 5 Flow" ("Channel to Cal")) -> (x-y=w767:u16)
            n409 = Index Array(array=w772) -> (element=w769:tag)  [unwired: 1 in]
            n410 = Format Into String(format string="%s/port1/line%d", w769, w767) -> (resulting string=w765:string)  [unwired: 2 in, 1 out]
            n411 = call-poly <vilib>:"DAQmx Create Virtual Channel.vi"("lines"=w765) -> ("task out"=w764:refnum<k21>)  [unwired: 13 in, 1 out]
            n412 = call-poly <vilib>:"DAQmx Write.vi"("task/channels in"=w764, "data"=TRUE) -> ()  [unwired: 11 in, 3 out]
          }
        }
      }
      frame "Start Cal" {
        w775 = T10."Enabled" ("Disabled")
        n413 = property on="Reading Value 1" class="DigNum (strict)"("DisabledEnum"=w775) -> ()  [unwired: 2 in, 2 out]
        n414 = property on="Cal Value 1" class="DigNum (strict)"("DisabledEnum"=w775) -> (error out=w776:errorcluster)  [unwired: 2 in, 1 out]
        n415 = property on="Confirm 1st Point" class="Bool"("DisabledEnum"=w775) -> ()  [unwired: 2 in, 2 out]
        n416 = property on="Cal Value 1" class="DigNum (strict)"(error in=w776, "Key Focus"=TRUE) -> ()  [unwired: 1 in, 2 out]
        n417 = Insert Into Array(array=w778, index=0, new element=string[] ["First Cal Point"]) -> (w779:string[])
      }
      frame "First Cal Point" {
        # "Handle Digital to Analog Conversion"
        n418 = Unbundle By Name(w790) -> ("Selected Chassis"=w788:tag, "Channel to Cal"=w782:T2, "Cal Unit"=w786:T1, "Rack Version"=w784:T5)
        n419 = call "DAQ Rack AI Read.vi"("Rack Version"=w784, "Cal Unit"=w786, "Channel to Cal"=w782, "Chassis"=w788) -> ("Lost Connection"=w785:bool, "Available?"=w787:bool, "Data"=w783:dbl)  [unwired: 5 in]
        n420 = case shown="\"RIO\"" w784 {
          tunnel: w783 -> [w795 w801]
          tunnel: w782 -> [w796 _]
          tunnel: [w794 w801] -> w781
          frame "RIO" {
            n421 = case shown="\"AI-22 Pos 1 Pressure\"..\"AI-33 Pos 6 Flow\"" w796 {
              tunnel: w795 -> [w797 w799]
              tunnel: [w797 w798] -> w794
              frame Default {
              }
              frame "AI-22 Pos 1 Pressure".."AI-33 Pos 6 Flow" {
                n422 = Divide(x=w799, y=13107.0) -> (x/y=w798:dbl)
              }
            }
          }
          frame Default {
          }
        }
        n423 = case shown="True" w787 {
          tunnel: w781 -> [_ w804]
          frame False {
          }
          frame True {
            n424 = call <vilib>:"Mean PtByPt.vi"("x"=w804, "sample length"="avg") -> ("mean"=→"Reading Value 1":dbl)  [unwired: 2 in, 1 out]
          }
        }
        n425 = case shown="False" w785 {
          tunnel: [string[] ["Main", "First Cal Point"] string[] ["End Cal"]] -> w791
          frame False {
          }
          frame True {
          }
        }
        n426 = Insert Into Array(array=w792, index=0, new element=w791) -> (w793:string[])
      }
      frame "Second Cal Point" {
        # "Handle Digital to Analog Conversion"
        n427 = Unbundle By Name(w816) -> ("Selected Chassis"=w814:tag, "Channel to Cal"=w809:T2, "Cal Unit"=w812:T1, "Rack Version"=w810:T5)
        n428 = call "DAQ Rack AI Read.vi"("Rack Version"=w810, "Cal Unit"=w812, "Channel to Cal"=w809, "Chassis"=w814) -> ("Lost Connection"=w811:bool, "Available?"=w813:bool, "Data"=w808:dbl)  [unwired: 5 in]
        n429 = case shown="\"RIO\"" w810 {
          tunnel: w808 -> [w821 w827]
          tunnel: w809 -> [w822 _]
          tunnel: [w820 w827] -> w807
          frame "RIO" {
            n430 = case shown="\"AI-22 Pos 1 Pressure\"..\"AI-33 Pos 6 Flow\"" w822 {
              tunnel: w821 -> [w823 w825]
              tunnel: [w823 w824] -> w820
              frame Default {
              }
              frame "AI-22 Pos 1 Pressure".."AI-33 Pos 6 Flow" {
                n431 = Divide(x=w825, y=13107.0) -> (x/y=w824:dbl)
              }
            }
          }
          frame Default {
          }
        }
        n432 = case shown="False" w811 {
          tunnel: [string[] ["Main", "Second Cal Point"] string[] ["End Cal"]] -> w819
          frame False {
          }
          frame True {
          }
        }
        n433 = case shown="True" w813 {
          tunnel: w807 -> [_ w830]
          frame False {
          }
          frame True {
            n434 = local read "avg"() -> (w831:i32)
            n435 = call <vilib>:"Mean PtByPt.vi"("x"=w830, "sample length"=w831) -> ("mean"=→"Reading Value 2":dbl)  [unwired: 2 in, 1 out]
          }
        }
        n436 = Insert Into Array(array=w818, index=0, new element=w819) -> (w817:string[])
      }
      frame "Third Cal Point" {
        # "Handle Digital to Analog Conversion"
        n437 = Unbundle By Name(w842) -> ("Selected Chassis"=w840:tag, "Channel to Cal"=w834:T2, "Cal Unit"=w838:T1, "Rack Version"=w835:T5)
        n438 = call "DAQ Rack AI Read.vi"("Rack Version"=w835, "Cal Unit"=w838, "Channel to Cal"=w834, "Chassis"=w840) -> ("Lost Connection"=w837:bool, "Available?"=w839:bool, "Data"=w836:dbl)  [unwired: 5 in]
        n439 = case shown="\"RIO\"" w835 {
          tunnel: w836 -> [w847 w853]
          tunnel: w834 -> [w848 _]
          tunnel: [w846 w853] -> w833
          frame "RIO" {
            n440 = case shown="\"AI-22 Pos 1 Pressure\"..\"AI-33 Pos 6 Flow\"" w848 {
              tunnel: w847 -> [w849 w851]
              tunnel: [w849 w850] -> w846
              frame Default {
              }
              frame "AI-22 Pos 1 Pressure".."AI-33 Pos 6 Flow" {
                n441 = Divide(x=w851, y=13107.0) -> (x/y=w850:dbl)
              }
            }
          }
          frame Default {
          }
        }
        n442 = case shown="False" w837 {
          tunnel: [string[] ["Main", "Third Cal Point"] string[] ["End Cal"]] -> w845
          frame False {
          }
          frame True {
          }
        }
        n443 = case shown="True" w839 {
          tunnel: w833 -> [_ w856]
          frame False {
          }
          frame True {
            n444 = local read "avg"() -> (w857:i32)
            n445 = call <vilib>:"Mean PtByPt.vi"("x"=w856, "sample length"=w857) -> ("mean"=→"Reading Value 3":dbl)  [unwired: 2 in, 1 out]
          }
        }
        n446 = Insert Into Array(array=w844, index=0, new element=w845) -> (w843:string[])
      }
      frame "Fourth Cal Point" {
        # "Handle Digital to Analog Conversion"
        n447 = Unbundle By Name(w868) -> ("Selected Chassis"=w866:tag, "Channel to Cal"=w860:T2, "Cal Unit"=w864:T1, "Rack Version"=w861:T5)
        n448 = call "DAQ Rack AI Read.vi"("Rack Version"=w861, "Cal Unit"=w864, "Channel to Cal"=w860, "Chassis"=w866) -> ("Lost Connection"=w863:bool, "Available?"=w865:bool, "Data"=w862:dbl)  [unwired: 5 in]
        n449 = case shown="\"RIO\"" w861 {
          tunnel: w862 -> [w873 w879]
          tunnel: w860 -> [w874 _]
          tunnel: [w872 w879] -> w859
          frame "RIO" {
            n450 = case shown="Default" w874 {
              tunnel: w873 -> [w875 w877]
              tunnel: [w875 w876] -> w872
              frame Default {
              }
              frame "AI-22 Pos 1 Pressure".."AI-33 Pos 6 Flow" {
                n451 = Divide(x=w877, y=13107.0) -> (x/y=w876:dbl)
              }
            }
          }
          frame Default {
          }
        }
        n452 = case shown="False" w863 {
          tunnel: [string[] ["Main", "Fourth Cal Point"] string[] ["End Cal"]] -> w871
          frame False {
          }
          frame True {
          }
        }
        n453 = case shown="True" w865 {
          tunnel: w859 -> [_ w883]
          frame False {
          }
          frame True {
            n454 = local read "avg"() -> (w884:i32)
            n455 = call <vilib>:"Mean PtByPt.vi"("x"=w883, "sample length"=w884) -> ("mean"=→"Reading Value 4":dbl)  [unwired: 2 in, 1 out]
          }
        }
        n456 = Insert Into Array(array=w870, index=0, new element=w871) -> (w869:string[])
      }
      frame "Final Cal Point" {
        # "Handle Digital to Analog Conversion"
        n457 = Unbundle By Name(w894) -> ("Selected Chassis"=w892:tag, "Channel to Cal"=w886:T2, "Cal Unit"=w890:T1, "Rack Version"=w887:T5)
        n458 = call "DAQ Rack AI Read.vi"("Rack Version"=w887, "Cal Unit"=w890, "Channel to Cal"=w886, "Chassis"=w892) -> ("Lost Connection"=w889:bool, "Available?"=w891:bool, "Data"=w888:dbl)  [unwired: 5 in]
        n459 = case shown="Default" w887 {
          tunnel: w888 -> [w899 w905]
          tunnel: w886 -> [w900 _]
          tunnel: [w898 w905] -> w885
          frame "RIO" {
            n460 = case shown="\"AI-22 Pos 1 Pressure\"..\"AI-33 Pos 6 Flow\"" w900 {
              tunnel: w899 -> [w901 w903]
              tunnel: [w901 w902] -> w898
              frame Default {
              }
              frame "AI-22 Pos 1 Pressure".."AI-33 Pos 6 Flow" {
                n461 = Divide(x=w903, y=13107.0) -> (x/y=w902:dbl)
              }
            }
          }
          frame Default {
          }
        }
        n462 = case shown="False" w889 {
          tunnel: [string[] ["Main", "Final Cal Point"] string[] ["End Cal"]] -> w897
          frame False {
          }
          frame True {
          }
        }
        n463 = case shown="False" w891 {
          tunnel: w885 -> [_ w909]
          frame False {
          }
          frame True {
            n464 = local read "avg"() -> (w910:i32)
            n465 = call <vilib>:"Mean PtByPt.vi"("x"=w909, "sample length"=w910) -> ("mean"=→"Reading Value 5":dbl)  [unwired: 2 in, 1 out]
          }
        }
        n466 = Insert Into Array(array=w896, index=0, new element=w897) -> (w895:string[])
      }
      frame "Calculate Coeffs" {
        w912 = T10."Enabled" ("Disabled")
        w911 = T10."Disabled and Grayed Out" ("Disabled")
        n467 = Unbundle By Name(w919) -> ("Channel to Cal"=w915:T2, "Cal Unit"=w918:T1, "Verification"=w917:bool, "Cal Log"=w916:string[][])
        n468 = case shown="False" w917 {
          tunnel: [w937 w964] -> w928
          tunnel: [w936 w963] -> w927
          tunnel: [w935 w962] -> w926
          tunnel: w918 -> [w934 w961]
          tunnel: w916 -> [_ w965]
          tunnel: w915 -> [_ w966]
          tunnel: [w933 w960] -> w914
          tunnel: [w932 w959] -> w913
          frame False {
            n469 = case shown="\"V\", \"Hz\", Default" w934 {
              tunnel: [w950 w957] -> w937
              tunnel: [w949 1.0] -> w936
              tunnel: [w948 w957] -> w935
              tunnel: [w939 w957] -> w933
              tunnel: [w938 w957] -> w932
              frame "V", "Hz", Default {
                n470 = local read "Reading Value 1"() -> (w953:dbl)
                n471 = local read "Reading Value 2"() -> (w952:dbl)
                n472 = local read "Reading Value 3"() -> (w951:dbl)
                n473 = local read "Reading Value 4"() -> (w941:dbl)
                n474 = local read "Reading Value 5"() -> (w940:dbl)
                n475 = Build Array("Cal Value 1", "Cal Value 2", "Cal Value 3", "Cal Value 4", "Cal Value 5") -> (w947:dbl[])
                n476 = Build Array(w953, w952, w951, w941, w940) -> (w946:dbl[])
                n477 = call <vilib>:"General Polynomial Fit Coefficients.vi"("Y"=w947, "polynomial order"=4, "X"=w946) -> ("Polynomial Coefficients"=w945:dbl[])  [unwired: 11 in, 1 out]
                n478 = Index Array(array=w945) -> (element #1=w950:dbl, element #2=w949:dbl, element #3=w948:dbl, element #4=w939:dbl, element #5=w938:dbl)  [unwired: 5 in]
              }
              frame "deg C" {
                w957 = 0.0
              }
            }
          }
          frame True {
            n479 = case shown="Default" w961 {
              selector: w961 -> [w969 _]
              tunnel: w966 -> [w985 _]
              tunnel: w965 -> [w977 _]
              tunnel: [w972 w991] -> w964
              tunnel: [w971 1.0 ("Label")] -> w963
              tunnel: [w970 w991] -> w962
              tunnel: [w968 w991] -> w960
              tunnel: [w967 w991] -> w959
              frame Default {
                n480 = Format Into String(w985) -> (resulting string=w982:string)  [unwired: 3 in, 1 out]
                n481 = Format Into String(w969) -> (resulting string=w978:string)  [unwired: 3 in, 1 out]
                n482 = Index Array(array=w977, index (col) #1=0 ("disabled index (col)"), index (col) #2=1 ("index (col)")) -> (element #1=w983:string[], element #2=w979:string[])  [unwired: 2 in]
                n483 = call-poly <userlib>:"Search Array__ogtk.vi"("Array"=w983, "Element Data"=w982) -> ("Indices of Elements"=w980:i32[])  [unwired: 7 in]
                n484 = for {
                  tunnel: w980 -> [w986] mode=indexing
                  tunnel: w979 -> [w990]
                  tunnel: w978 -> [w988]
                  tunnel: [w986] -> w976
                  stop <- w987 stop-if-true
                  n485 = Index Array(array=w990, index=w986) -> (element=w989:string)
                  n486 = Equal?(x=w988, y=w989) -> (x = y?=w987:bool)
                }
                n487 = Index Array(array=w977, index (row)=w976) -> (element=w975:string[])  [unwired: 1 in]
                n488 = Fract/Exp String To Number(string=w975) -> (number=w974:dbl[])  [unwired: 3 in, 1 out]
                n489 = Index Array(array=w974, index #1=12 ("index")) -> (element #1=w972:dbl, element #2=w971:dbl, element #3=w970:dbl, element #4=w968:dbl, element #5=w967:dbl)  [unwired: 4 in]
              }
              frame "deg C" {
                w991 = 0.0 ("Label")
              }
            }
          }
        }
        "a0" <- w928
        "a2" <- w926
        "a1" <- w927
        "a4" <- w913
        "a3" <- w914
        n490 = property on="Reading Value 5" class="DigNum (strict)"("DisabledEnum"=w911) -> ()  [unwired: 2 in, 2 out]
        n491 = property on="Cal Value 5" class="DigNum (strict)"("DisabledEnum"=w911) -> ()  [unwired: 2 in, 2 out]
        n492 = property on="Confirm 5th Point" class="Bool"("DisabledEnum"=w911) -> ()  [unwired: 2 in, 2 out]
        n493 = property on="Cal Table" class="Tbl (strict)"("DisabledEnum"=w911) -> ()  [unwired: 2 in, 2 out]
        n494 = property on="Save Cal" class="Bool"("DisabledEnum"=T10."Enabled" ("Disabled")) -> ()  [unwired: 2 in, 2 out]
        n495 = property on="Verify Tab" class="TabCtl (strict)"("Visible"=TRUE) -> (error out=w923:errorcluster)  [unwired: 2 in, 1 out]
        n496 = property on="Verify Table" class="Tbl (strict)"(error in=w923, "Key Focus"=TRUE, "EditPos"=T11 {"Row"=0, "Column"=1} ("Active Cell:Active Cell")) -> ()  [unwired: 1 in, 2 out]
        n497 = Insert Into Array(array=w929, index=0, new element=string[] ["Cal Review"]) -> (w930:string[])
        n498 = property on="f(x)" class="DigNum (strict)"("DisabledEnum"=w912) -> ()  [unwired: 2 in, 2 out]
        n499 = property on="a0" class="DigNum (strict)"("DisabledEnum"=w912) -> ()  [unwired: 2 in, 2 out]
        n500 = property on="a1" class="DigNum (strict)"("DisabledEnum"=w912) -> ()  [unwired: 2 in, 2 out]
        n501 = property on="x" class="DigNum (strict)"("DisabledEnum"=w912) -> ()  [unwired: 2 in, 2 out]
        n502 = property on="a2" class="DigNum (strict)"("DisabledEnum"=w912) -> ()  [unwired: 2 in, 2 out]
        n503 = property on="a3" class="DigNum (strict)"("DisabledEnum"=w912) -> ()  [unwired: 2 in, 2 out]
        n504 = property on="a4" class="DigNum (strict)"("DisabledEnum"=w912) -> ()  [unwired: 2 in, 2 out]
      }
      frame "Cal Review" {
        # "Handle Digital to Analog Conversion"
        n505 = property on="Verify Table" class="Tbl (strict)"() -> ("EditPos"=w1025:T11)  [unwired: 2 in, 2 out]
        n506 = Unbundle By Name(w1009) -> ("Init Mean"=w1010:bool, "Selected Chassis"=w1012:tag, "Channel to Cal"=w997:T2, "Cal Unit"=w998:T1, "Rack Version"=w994:T5, "Auto"=w1007:bool, "Verify Table"=w1011:string[][])
        n507 = Unbundle(w1025) -> ("Row"=w1023:i32)  [unwired: 1 out]
        n508 = Greater Or Equal To 0?(x=w1023) -> (x >= 0?=w1024:bool)
        n509 = Index Array(array=w1011, index (row)=w1023, index (col)=0 ("disabled index (col)")) -> (element=w1015:string)
        n510 = Fract/Exp String To Number(string=w1015) -> (number=w1001:dbl)  [unwired: 3 in, 1 out]
        n511 = case shown="True" w1024 {
          tunnel: w1023 -> [_ w1053]
          frame False {
          }
          frame True {
            "Row" <- w1053
          }
        }
        n512 = call "DAQ Rack AI Read.vi"("Rack Version"=w994, "Cal Unit"=w998, "Channel to Cal"=w997, "Chassis"=w1012) -> ("Lost Connection"=w993:bool, "Available?"=w999:bool, "Data"=w996:dbl)  [unwired: 5 in]
        n513 = Increment(x=w1001) -> (x+1=w1017:dbl)
        n514 = case shown="\"RIO\"" w994 {
          tunnel: w996 -> [w1031 w1037]
          tunnel: w997 -> [w1032 _]
          tunnel: [w1030 w1037] -> w995
          frame "RIO" {
            n515 = case shown="\"AI-22 Pos 1 Pressure\"..\"AI-33 Pos 6 Flow\"" w1032 {
              tunnel: w1031 -> [w1033 w1035]
              tunnel: [w1033 w1034] -> w1030
              frame Default {
              }
              frame "AI-22 Pos 1 Pressure".."AI-33 Pos 6 Flow" {
                n516 = Divide(x=w1035, y=13107.0) -> (x/y=w1034:dbl)
              }
            }
          }
          frame Default {
          }
        }
        n517 = Empty String/Path?(string/path=w1015) -> (empty?=w1006:bool)
        n518 = Not(x=w1006) -> (.not. x?=w1018:bool)
        n519 = case shown="True" w999 {
          tunnel: w995 -> [_ w1046]
          tunnel: w1010 -> [_ w1045]
          tunnel: [w1040 w1044] -> w1002
          frame False {
            n520 = local read "f(x)"() -> (w1040:dbl)
          }
          frame True {
            n521 = local read "avg"() -> (w1043:i32)
            n522 = call <vilib>:"Mean PtByPt.vi"("x"=w1046, "sample length"=w1043, "initialize"=w1045) -> ("mean"=w1051:dbl)  [unwired: 1 in, 1 out]
            "x" <- w1051
            n523 = local read "a0"() -> (w1050:dbl)
            n524 = local read "a1"() -> (w1049:dbl)
            n525 = local read "a2"() -> (w1048:dbl)
            n526 = local read "a3"() -> (w1042:dbl)
            n527 = local read "a4"() -> (w1041:dbl)
            n528 = Build Array(w1050, w1049, w1048, w1042, w1041) -> (w1047:dbl[])
            n529 = call <vilib>:"1D Polynomial Evaluation PtByPt.vi"("Coefficients: a"=w1047, "x"=w1051) -> ("y"=w1044:dbl)
            "f(x)" <- w1044
          }
        }
        n530 = Increment(x=w1002) -> (x+1=w1016:dbl)
        n531 = Subtract(x=w1016, y=w1017) -> (x-y=w1003:dbl)
        n532 = Divide(x=w1003, y=w1016) -> (x/y=w1021:dbl)
        n533 = Absolute Value(x=w1021) -> (abs(x)=w1000:dbl)
        n534 = Less?(x=w1000, y=0.1) -> (x < y?=w1019:bool)
        n535 = Compound Arithmetic op=AND(w1007, w1019, w1018) -> (w1014:bool)
        n536 = call "Reading Delay.vi"("Delay"="ms", "In Range"=w1014) -> ("Take Reading"=w1005:bool)  [unwired: 9 in]
        n537 = case shown="False" w993 {
          tunnel: [string[] ["Main", "Cal Review"] string[] ["End Cal"]] -> w1029
          frame False {
          }
          frame True {
          }
        }
        n538 = case shown="True" w1005 {
          selector: w1005 -> [_ w1052]
          frame False {
          }
          frame True {
            n539 = property on="Verify Read" class="Bool (strict)"("Val(Sgnl)"=w1052) -> ()  [unwired: 2 in, 2 out]
          }
        }
        n540 = Insert Into Array(array=w1027, index=0, new element=w1029) -> (w1028:string[])
        n541 = Bundle By Name(cluster=w1009, "Init Mean"=FALSE) -> (w1004:T9)
      }
      frame "Save Cal" {
        w1100 = u16 4 ("y")
        n542 = Unbundle By Name(w1075) -> ("Cal File Path"=w1085:path, "Cal Log Header"=w1107:string[], "Cal Log"=w1071:string[][], "Channel to Cal"=w1083:T2, "Cal Unit"=w1084:T1, "Verification"=w1074:bool, "Verify Table"=w1086:string[][])
        n543 = local read "Reading Value 1"() -> (w1068:dbl)
        n544 = local read "Reading Value 2"() -> (w1066:dbl)
        n545 = local read "Reading Value 3"() -> (w1064:dbl)
        n546 = local read "Reading Value 4"() -> (w1062:dbl)
        n547 = local read "Reading Value 5"() -> (w1060:dbl)
        n548 = local read "Cal Value 1"() -> (w1067:dbl)
        n549 = local read "Cal Value 2"() -> (w1065:dbl)
        n550 = local read "Cal Value 3"() -> (w1063:dbl)
        n551 = local read "Cal Value 4"() -> (w1061:dbl)
        n552 = local read "Cal Value 5"() -> (w1059:dbl)
        n553 = local read "a0"() -> (w1058:dbl)
        n554 = local read "a1"() -> (w1057:dbl)
        n555 = local read "a2"() -> (w1056:dbl)
        n556 = local read "a3"() -> (w1055:dbl)
        n557 = local read "a4"() -> (w1054:dbl)
        n558 = Build Array(w1068, w1067, w1066, w1065, w1064, w1063, w1062, w1061, w1060, w1059, w1058, w1057, w1056, w1055, w1054) -> (w1113:dbl[])
        n559 = Format Into String(w1083) -> (resulting string=w1079:string)  [unwired: 3 in, 1 out]
        n560 = Format Into String(w1084) -> (resulting string=w1076:string)  [unwired: 3 in, 1 out]
        n561 = Index Array(array=w1071, index (col) #1=0 ("disabled index (col)"), index (col) #2=1 ("index (col)")) -> (element #1=w1080:string[], element #2=w1078:string[])  [unwired: 2 in]
        n562 = Search 1D Array(1D array=w1080, element=w1079) -> (index of element=w1077:i32)  [unwired: 1 in]
        n563 = Search 1D Array(1D array=w1078, element=w1076, start index (0)=w1077) -> (index of element=w1070:i32)
        n564 = Index Array(array=w1086, index (col) #1=0 ("disabled index (col)"), index (col) #2=1 ("disabled index (col)")) -> (element #1=w1090:string[], element #2=w1089:string[])  [unwired: 2 in]
        n565 = Index Array(array=w1071, index (row)=w1070) -> (element=w1069:string[])  [unwired: 1 in]
        n566 = Format Date/Time String(time format string (%c)="%d%b%y %I:%M:%S %p") -> (date/time string=w1111:string)  [unwired: 2 in]
        n567 = Interleave 1D Arrays(w1090, w1089) -> (w1088:string[])
        n568 = To Upper Case(1:w1111) -> (0:w1073:string)
        n569 = case shown="True" w1074 {
          tunnel: w1113 -> [w1120 _]
          tunnel: [w1118 w1122] -> w1112
          tunnel: [w1117 w1121] -> w1072
          tunnel: w1073 -> [w1117 _]
          tunnel: w1069 -> [_ w1124]
          frame False {
            n570 = Number To Fractional String(number=w1120, precision (6)=i16 4) -> (F-format string=w1118:string[])  [unwired: 2 in]
          }
          frame True {
            n571 = Array Subset(array=w1124, index=2, length=9) -> (w1122:string[])
            n572 = Index Array(array=w1124, index=11) -> (element=w1121:string)
          }
        }
        n573 = Build Array (concatenate)(w1079, w1076, w1112, w1072, w1088) -> (w1109:string[])
        n574 = Greater?(x=w1070, y=w1100) -> (0:w1099:bool)
        n575 = Subtract(x=w1070, y=w1100) -> (x-y=w1098:i32)
        n576 = Bundle(cluster=T11 {"Row"=0, "Column"=0} ("Active Cell:Active Cell"), "Row"=w1070, "Column"=-2) -> (w1101:T11)
        n577 = Select(t=w1098, s=w1099, f=u16 0 ("y")) -> (s? t:f=w1095:i32)
        n578 = Replace Array Subset(array=w1071, new element=w1109, index (row)=w1070) -> (w1106:string[][])  [unwired: 1 in]
        n579 = Bundle(cluster=T11 {"Row"=0, "Column"=0} ("Active Cell:Active Cell"), "Row"=w1095, "Column"=0) -> (w1094:T11)
        n580 = Build Array (concatenate)(w1107, w1106) -> (w1105:string[][])
        n581 = Insert Into Array(array=w1114, index=0, new element=string[] ["Write to Excel", "Load Cal File", "End Cal", "Increment Channel"]) -> (w1115:string[])
        n582 = property on="Cal Table" class="Tbl (strict)"("Active Cell"=w1101, "Cell BG Color"=u32 16775793, "Index Values"=w1094) -> ()  [unwired: 2 in, 2 out]
        n583 = call-poly <vilib>:"Write To Spreadsheet File.vi"("delimiter (\\t)"="," ("delimiter (\\t)"), "2D data"=w1105, "file path (dialog if empty)"=w1085) -> ()  [unwired: 5 in, 1 out]
      }
      frame "Calc Dev" {
        n584 = Unbundle By Name(w1134) -> ("Verify Table"=w1131:string[][], "Cal Unit"=w1128:T1, "Rack Version"=w1127:T5, "Verify Table Ref"=w1130:refnum<vi>)
        n585 = call "Calc Dev (DAQ Rack).vi"("Verify Table IN"=w1131, "Units"=w1128, "Rack Version"=w1127, "Dev Table 1 Ref"=w1130) -> ("Verify Table OUT"=w1129:string[][])  [unwired: 15 in]
        n586 = local write "Verify Table"(w1129) -> ()
        n587 = Bundle By Name(cluster=w1134, "Verify Table"=w1129) -> (w1133:T9)
        n588 = Insert Into Array(array=w1136, index=0, new element=string[] []) -> (w1135:string[])
      }
      frame "Write to Excel" {
        n589 = Unbundle By Name(w1145) -> ("Cal Spreadsheet Path"=w1149:path, "Verify Table"=w1142:string[][], "Channel to Cal"=w1139:T2, "Cal Unit"=w1138:T1)
        n590 = flat-sequence {
          tunnel: w1149 -> [w1156]
          tunnel: [w1156] -> w1150
          tunnel: [w1153] -> w1143
          tunnel: w1142 -> [w1153]
          tunnel: [w1152] -> w1141
          tunnel: w1139 -> [w1152]
          tunnel: [w1151] -> w1140
          tunnel: w1138 -> [w1151]
          tunnel: w1150 -> [w1160]
          tunnel: w1143 -> [w1159]
          tunnel: w1141 -> [w1158]
          tunnel: w1140 -> [w1157]
          frame #0 {
            n591 = property on="Main Tab" class="TabCtl (strict)"("DisabledEnum"=T10."Disabled" ("Disabled")) -> ()  [unwired: 2 in, 2 out]
            n592 = property on="Load Indicator Tab" class="TabCtl (strict)"("Visible"=TRUE) -> ()  [unwired: 2 in, 2 out]
          }
          frame #1 {
            n593 = call "Write DAQ Rack Data.vi"("Cal Unit"=w1157, "Channel to Cal"=w1158, "Verify Table"=w1159, "Cal Path"=w1160) -> ()  [unwired: 8 in]
          }
          frame #2 {
            n594 = property on="Main Tab" class="TabCtl (strict)"("DisabledEnum"=T10."Enabled" ("Disabled")) -> ()  [unwired: 2 in, 2 out]
            n595 = property on="Load Indicator Tab" class="TabCtl (strict)"("Visible"=FALSE) -> ()  [unwired: 2 in, 2 out]
          }
        }
        n596 = Insert Into Array(array=w1147, index=0, new element=string[] ["Recolor Tables"]) -> (w1146:string[])
      }
      frame "Recolor Tables" {
        n597 = Unbundle By Name(w1167) -> ("Verify Table Ref"=w1166:refnum<vi>)
        n598 = property on="Property Node" class="Tbl (strict)"(reference=w1166, "Active Cell"=T11 {"Row"=-2, "Column"=-2} ("Active Cell:Active Cell"), "Cell BG Color"=u32 15527148) -> (reference out=w1163:refnum<vi>)  [unwired: 1 in, 1 out]
        n599 = property on="Property Node" class="Tbl (strict)"(reference=w1163, "Active Cell"=T11 {"Row"=-2, "Column"=1} ("Active Cell:Active Cell"), "Cell BG Color"=u32 16448250) -> ()  [unwired: 1 in, 2 out]
      }
      frame "End Cal" {
        w1174 = 0 items=["one channel for each line", "one channel for all lines"] ("line grouping")
        w1193 = T10."Disabled and Grayed Out" ("Disabled")
        w1194 = 0.0 ("Reading Value 1")
        w1187 = FALSE ("Visible")
        # "Turn off all parasitic relays."
        n600 = Unbundle By Name(w1192) -> ("Selected Chassis"=w1180:tag, "Cal Spreadsheet Path"=w1191:path)
        n601 = property on="Output Tab" class="TabCtl (strict)"("Visible"=w1187) -> ()  [unwired: 2 in, 2 out]
        n602 = property on="Header Tab" class="TabCtl (strict)"("Visible"=w1187) -> ()  [unwired: 2 in, 2 out]
        n603 = property on="Load Indicator Tab" class="TabCtl (strict)"("Visible"=w1187) -> ()  [unwired: 2 in, 2 out]
        n604 = property on="Cancel Cal" class="Bool (strict)"("Value"=FALSE ("Cancel Cal")) -> ()  [unwired: 2 in, 2 out]
        n605 = property on="Main Tab" class="TabCtl (strict)"("DisabledEnum"=T10."Enabled" ("Disabled")) -> ()  [unwired: 2 in, 2 out]
        n606 = property on="Header" class="Bool"("DisabledEnum"=T10."Enabled" ("Disabled")) -> ()  [unwired: 2 in, 2 out]
        n607 = Empty String/Path?(string/path=w1191) -> (empty?=w1190:bool)
        n608 = Select(t=2, s=w1190, f=0) -> (s? t:f=w1171:i32)
        n609 = property on="Tank IP:" class="Str"("DisabledEnum"=w1171) -> ()  [unwired: 2 in, 2 out]
        n610 = property on="Channel to Cal" class="Enum (strict)"("DisabledEnum"=w1171) -> ()  [unwired: 2 in, 2 out]
        n611 = property on="Start Cal" class="Bool"("DisabledEnum"=w1171) -> ()  [unwired: 2 in, 2 out]
        n612 = property on="Cal Unit" class="Enum (strict)"("DisabledEnum"=w1171) -> ()  [unwired: 2 in, 2 out]
        n613 = property on="View Spreadsheet" class="Bool"("DisabledEnum"=w1171) -> ()  [unwired: 2 in, 2 out]
        n614 = property on="Start Verification" class="Bool"("DisabledEnum"=w1171) -> ()  [unwired: 2 in, 2 out]
        n615 = local write "Reading Value 1"(w1194) -> ()
        n616 = local write "Reading Value 2"(w1194) -> ()
        n617 = local write "Reading Value 3"(w1194) -> ()
        n618 = local write "Cal Value 1"(w1194) -> ()
        n619 = local write "Cal Value 2"(w1194) -> ()
        n620 = local write "Cal Value 3"(w1194) -> ()
        n621 = local write "a0"(w1194) -> ()
        n622 = local write "a1"(w1194) -> ()
        n623 = local write "a2"(w1194) -> ()
        n624 = property on="Header OK" class="Bool"("DisabledEnum"=w1193) -> ()  [unwired: 2 in, 2 out]
        n625 = property on="Header Cancel" class="Bool"("DisabledEnum"=w1193) -> ()  [unwired: 2 in, 2 out]
        n626 = property class="DAQmx Device"("Active Device"=w1180) -> (error out=w1175:errorcluster, "Chassis.ModuleDevNames"=w1183:tag[])  [unwired: 2 in, 1 out]
        n627 = call "TCP Data Stream PC.vi"("Mode"=TCP_Data_Stream_Mode_(PC)."Close") -> ()  [unwired: 15 in, 4 out]
        n628 = Index Array(array=w1183) -> (element=w1181:tag)  [unwired: 1 in]
        n629 = Format Into String(format string="%s/port1/line0:15", w1181) -> (resulting string=w1178:string)  [unwired: 2 in, 1 out]
        n630 = call-poly <vilib>:"DAQmx Create Virtual Channel.vi"("lines"=w1178, "line grouping"=w1174, "error in"=w1175) -> ("task out"=w1177:refnum<k21>, "error out"=w1176:errorcluster)  [unwired: 11 in]
        n631 = Insert Into Array(array=w1197, index=0, new element=string[] ["Recolor Tables", "Init Cal", "Button State"]) -> (w1198:string[])
        n632 = call-poly "DAQmx Write (Multi-Chan Multi-Samp 1D Wfm).vi"("task/channels in"=w1177, "data"=bool[] [FALSE, FALSE, FALSE, FALSE, FALSE, FALSE, FALSE, FALSE, FALSE, FALSE, FALSE, FALSE, FALSE, FALSE, FALSE, FALSE], "error in"=w1176) -> ("error out"=w1179:errorcluster)  [unwired: 10 in, 2 out]
        n633 = call <vilib>:"Clear Errors.vi"("error in (no error)"=w1179) -> ()  [unwired: 6 in, 1 out]
      }
      frame "Increment Channel" {
        n634 = Unbundle By Name(w1201) -> ("Channel to Cal"=w1200:T2)
        n635 = Increment(x=w1200) -> (x+1=w1199:T2)
        n636 = Bundle By Name(cluster=w1201, "Channel to Cal"=w1199) -> (w1202:T9)
        n637 = local write "Channel to Cal"(w1199) -> ()
      }
      frame "Exit" {
      }
    }
  }
